vi "CPU_core.vi"(11 "registers":T1 {"P" format="%08b"; "PC" format="%04x"; "SP" format="%02x"; "Y" format="%02x"; "X" format="%02x"; "A" format="%02x"}) -> (1 "clock ticks":u32, 2 "error":bool, 3 "registers":T1 {"P" format="%08b"; "PC" format="%04x"; "SP" format="%02x"; "Y" format="%02x"; "X" format="%02x"; "A" format="%02x"})   [LabVIEW 2018]
uses:
  CPU_registers.ctl
panel:
  # "This 6502 CPU core implements the full set of documented instructions,\ncovering arithmetic (ADC, SBC), logic (AND, ORA, EOR, BIT), shifts and rotates\n(ASL, LSR, ROL, ROR), comparisons (CMP, CPX, CPY), increments/decrements,\nbranches (BPL, BMI, BVC, BVS, BCC, BCS, BNE, BEQ), stack operations (PHA, PLA,\nPHP, PLP, RTS, RTI, BRK, JSR), transfers (TAX, TXA, TAY, TYA, TSX, TXS),\nand memory access (LDA, STA, LDX, STX, LDY, STY) across all addressing modes."
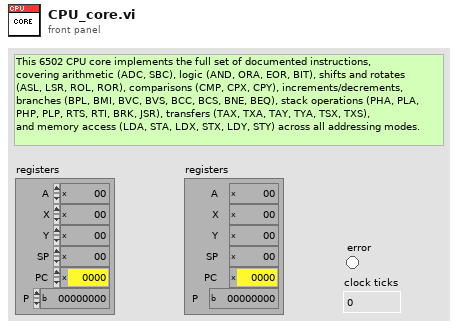
[diagram p1: front panel]
types:
  T1 = typedef "CPU_registers.ctl" = cluster{"A":u8, "X":u8, "Y":u8, "SP":u8, "PC":u16, "P":u8}
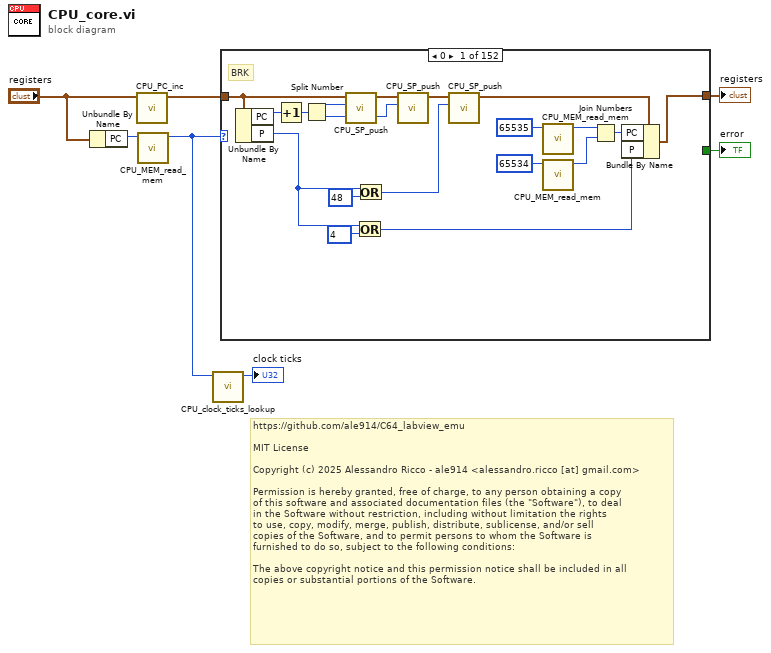
[diagram p0: block diagram]
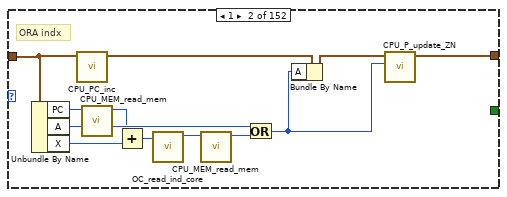
[diagram p2: hidden frame]
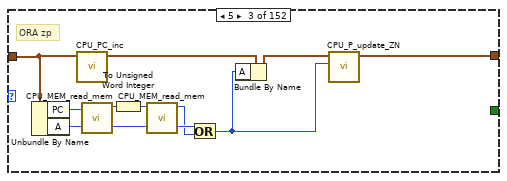
[diagram p3: hidden frame]
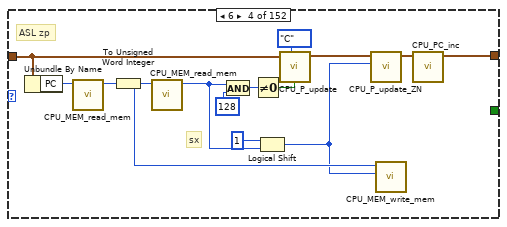
[diagram p4: hidden frame]
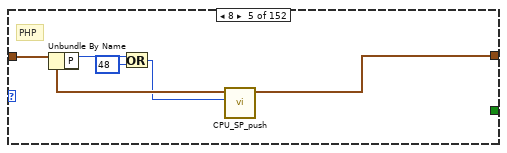
[diagram p5: hidden frame]
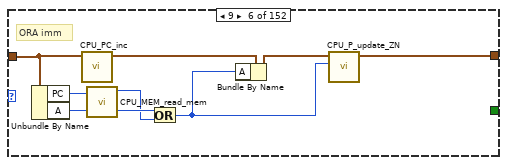
[diagram p6: hidden frame]
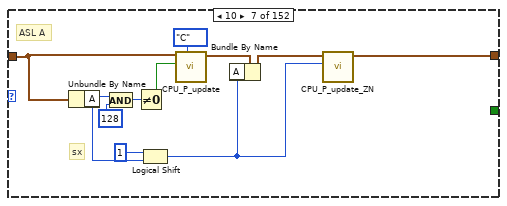
[diagram p7: hidden frame]
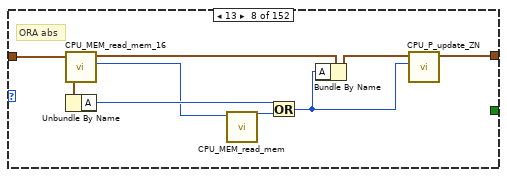
[diagram p8: hidden frame]
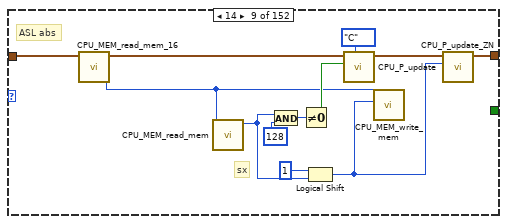
[diagram p9: hidden frame]
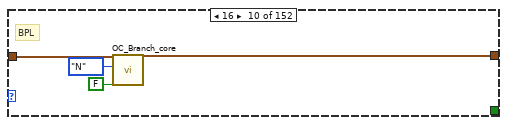
[diagram p10: hidden frame]
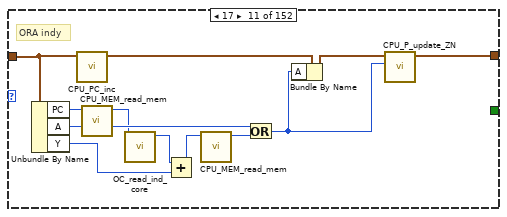
[diagram p11: hidden frame]
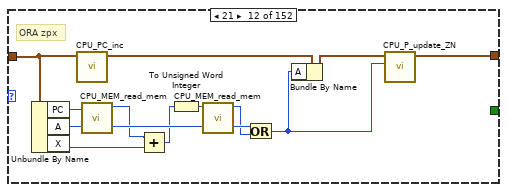
[diagram p12: hidden frame]
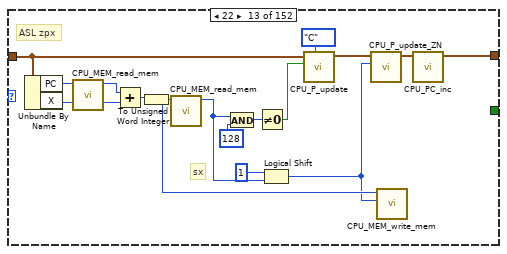
[diagram p13: hidden frame]
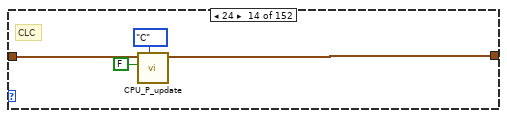
[diagram p14: hidden frame]
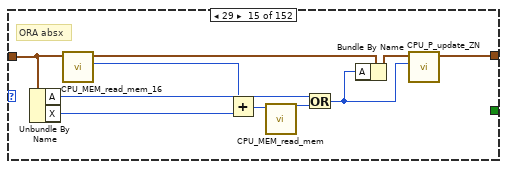
[diagram p15: hidden frame]
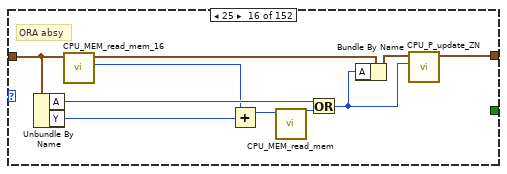
[diagram p16: hidden frame]
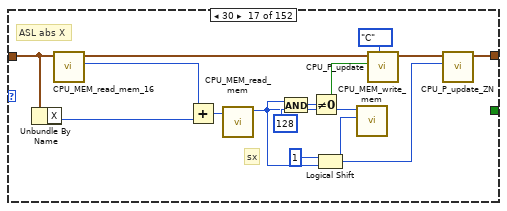
[diagram p17: hidden frame]
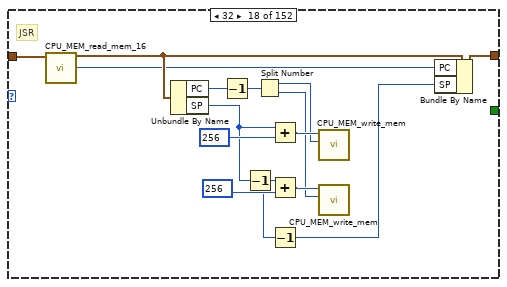
[diagram p18: hidden frame]
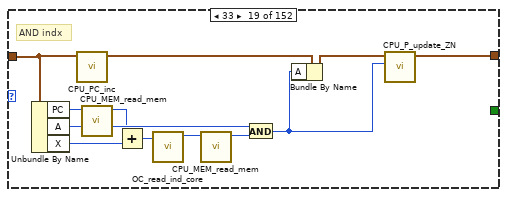
[diagram p19: hidden frame]
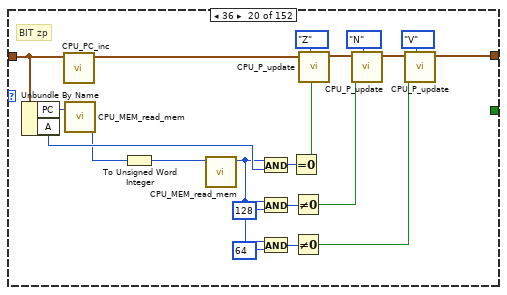
[diagram p20: hidden frame]
diagram:
  # "https://github.com/ale914/C64_labview_emu\n\nMIT License\n\nCopyright (c) 2025 Alessandro Ricco - ale914 <alessandro.ricco [at] gmail.com>\n\nPermission is hereby granted, free of charge, to any person obtaining a copy\nof this software and associated documentation files (the \"Software\"), to deal\nin the Software without restriction, including without limitation the rights\nto use, copy, modify, merge, publish, distribute, sublicense, and/or sell\ncopies of the Software, and to permit persons to whom the Software is\nfurnished to do so, subject to the following conditions:\n\nThe above copyright notice and this permission notice shall be included in all\ncopies or substantial portions of the Software."
  n1 = Unbundle By Name("registers") -> ("PC"=w4:u16)
  n2 = call "CPU_PC_inc.vi"("registers"="registers") -> ("registers"=w7:T1)  [unwired: 10 in]
  n3 = call "CPU_MEM_read_mem.vi"("address"=w4) -> ("value out"=w5:u8)  [unwired: 10 in]
  n4 = call "CPU_clock_ticks_lookup.vi"("opcode"=w5) -> ("clock ticks"=→"clock ticks":u32)  [unwired: 10 in]
  n5 = case shown="0" w5 {
    selector: w5 -> [_ _ _ _ _ _ _ _ _ _ _ _ _ _ _ _ _ _ _ _ _ _ _ _ _ _ _ _ _ _ _ _ _ _ _ _ _ _ _ _ _ _ _ _ _ _ _ _ _ _ _ _ _ _ _ _ _ _ _ _ _ _ _ _ _ _ _ _ _ _ _ _ _ _ _ _ _ _ _ _ _ _ _ _ _ _ _ _ _ _ _ _ _ _ _ _ _ _ _ _ _ _ _ _ _ _ _ _ _ _ _ _ _ _ _ _ _ _ _ _ _ _ _ _ _ _ _ _ _ _ _ _ _ _ _ _ _ _ _ _ _ _ _ _ _ _ _ _ _ _ _ w1390]
    tunnel: w7 -> [w14 w37 w46 w51 w65 w68 w85 w89 w97 w108 w121 w132 w140 w152 w157 w167 w177 w191 w214 w235 w244 w249 w268 w274 w284 w300 w319 w327 w343 w356 w367 w375 w394 w397 w407 w417 w440 w453 w462 w468 w480 w482 w499 w503 w507 w515 w526 w539 w550 w559 w572 w575 w585 w595 w610 w628 w634 w643 w647 w668 w674 w677 w696 w704 w709 w716 w723 w741 w752 w758 w779 w782 w808 w813 w819 w825 w831 w835 w838 w842 w846 w849 w859 w866 w874 w882 w887 w890 w896 w899 w907 w917 w923 w931 w939 w947 w952 w957 w962 w965 w971 w977 w982 w993 w1003 w1013 w1023 w1028 w1031 w1040 w1043 w1051 w1059 w1065 w1087 w1099 w1111 w1115 w1126 w1127 w1141 w1144 w1154 w1164 w1170 w1185 w1199 w1206 w1213 w1220 w1230 w1242 w1249 w1267 w1278 w1285 w1294 w1296 w1309 w1313 w1315 w1318 w1328 w1333 w1340 w1347 w1354 w1363 w1367 w1376 w1381 w1388]
    tunnel: [w23 w34 w43 w62 w64 w71 w78 w92 w101 w107 w118 w129 w150 w151 w162 w172 w183 w203 w211 w231 w241 w265 w273 w277 w282 w313 w322 w328 w342 w353 w364 w390 w391 w402 w412 w420 w441 w450 w459 w478 w479 w485 w493 w504 w510 w519 w525 w536 w547 w568 w569 w580 w590 w601 w609 w621 w632 w641 w665 w669 w672 w680 w699 w706 w713 w720 w727 w740 w749 w775 w776 w788 w803 w811 w817 w823 w827 w832 w837 w841 w845 w848 w854 w864 w872 w880 w884 w889 w894 w898 w904 w915 w920 w929 w937 w945 w949 w954 w959 w967 w973 w979 w981 w991 w1001 w1011 w1021 w1025 w1035 w1037 w1047 w1055 w1063 w1068 w1081 w1093 w1105 w1113 w1122 w1130 w1137 w1147 w1157 w1168 w1169 w1179 w1193 w1204 w1212 w1227 w1235 w1248 w1252 w1260 w1272 w1283 w1292 w1304 w1305 w1311 w1315 w1321 w1330 w1337 w1344 w1349 w1353 w1360 w1374 w1375 w1383 w1388] -> w3
    tunnel: [_ _ _ _ _ _ _ _ _ _ _ _ _ _ _ _ _ _ _ _ _ _ _ _ _ _ _ _ _ _ _ _ _ _ _ _ _ _ _ _ _ _ _ _ _ _ _ _ _ _ _ _ _ _ _ _ _ _ _ _ _ _ _ _ _ _ _ _ _ _ _ _ _ _ _ _ _ _ _ _ _ _ _ _ _ _ _ _ _ _ _ _ _ _ _ _ _ _ _ _ _ _ _ _ _ _ _ _ _ _ _ _ _ _ _ _ _ _ _ _ _ _ _ _ _ _ _ _ _ _ _ _ _ _ _ _ _ _ _ _ _ _ _ _ _ _ _ _ _ _ _ TRUE] -> w2
    frame 0 {
      # "BRK"
      n6 = Unbundle By Name(w14) -> ("PC"=w26:u16, "P"=w16:u8)
      n7 = Increment(x=w26) -> (x+1=w25:u16)
      n8 = Split Number(x=w25) -> (hi(x)=w13:u8, lo(x)=w11:u8)
      n9 = call "CPU_SP_push.vi"("value"=w13, "registers"=w14) -> ("registers"=w12:T1)  [unwired: 9 in]
      n10 = Or(x=w16, y=u8 4) -> (x .or. y?=w15:u8)
      n11 = Or(x=w16, y=u8 48) -> (x .or. y?=w9:u8)
      n12 = call "CPU_SP_push.vi"("value"=w11, "registers"=w12) -> ("registers"=w10:T1)  [unwired: 9 in]
      n13 = call "CPU_SP_push.vi"("value"=w9, "registers"=w10) -> ("registers"=w8:T1)  [unwired: 9 in]
      n14 = call "CPU_MEM_read_mem.vi"("address"=u16 65535) -> ("value out"=w20:u8)  [unwired: 10 in]
      n15 = call "CPU_MEM_read_mem.vi"("address"=u16 65534) -> ("value out"=w19:u8)  [unwired: 10 in]
      n16 = Join Numbers(hi=w20, lo=w19) -> ((hi.lo)=w18:u16)
      n17 = Bundle By Name(cluster=w8, "PC"=w18, "P"=w15) -> (w23:T1)
    }
    frame 1 {
      # "ORA indx"
      n18 = Unbundle By Name(w37) -> ("PC"=w31:u16, "A"=w36:u8, "X"=w32:u8)
      n19 = call "CPU_PC_inc.vi"("registers"=w37) -> ("registers"=w38:T1)  [unwired: 10 in]
      n20 = call "CPU_MEM_read_mem.vi"("address"=w31) -> ("value out"=w30:u8)  [unwired: 10 in]
      n21 = Add(x=w30, y=w32) -> (x+y=w29:u8)
      n22 = call "OC_read_ind_core.vi"("base"=w29) -> ("addr"=w28:u16)  [unwired: 10 in]
      n23 = call "CPU_MEM_read_mem.vi"("address"=w28) -> ("value out"=w27:u8)  [unwired: 10 in]
      n24 = Or(x=w36, y=w27) -> (x .or. y?=w33:u8)
      n25 = Bundle By Name(cluster=w38, "A"=w33) -> (w35:T1)
      n26 = call "CPU_P_update_ZN.vi"("value"=w33, "registers"=w35) -> ("registers"=w34:T1)  [unwired: 9 in]
    }
    frame 5 {
      # "ORA zp"
      n27 = Unbundle By Name(w46) -> ("PC"=w47:u16, "A"=w45:u8)
      n28 = call "CPU_PC_inc.vi"("registers"=w46) -> ("registers"=w48:T1)  [unwired: 10 in]
      n29 = call "CPU_MEM_read_mem.vi"("address"=w47) -> ("value out"=w40:u8)  [unwired: 10 in]
      n30 = To Unsigned Word Integer(number=w40) -> (unsigned 16bit integer=w39:u16)
      n31 = call "CPU_MEM_read_mem.vi"("address"=w39) -> ("value out"=w41:u8)  [unwired: 10 in]
      n32 = Or(x=w45, y=w41) -> (x .or. y?=w42:u8)
      n33 = Bundle By Name(cluster=w48, "A"=w42) -> (w44:T1)
      n34 = call "CPU_P_update_ZN.vi"("value"=w42, "registers"=w44) -> ("registers"=w43:T1)  [unwired: 9 in]
    }
    frame 6 {
      # "sx"
      # "ASL zp"
      n35 = Unbundle By Name(w51) -> ("PC"=w54:u16)
      n36 = call "CPU_MEM_read_mem.vi"("address"=w54) -> ("value out"=w53:u8)  [unwired: 10 in]
      n37 = To Unsigned Word Integer(number=w53) -> (unsigned 16bit integer=w50:u16)
      n38 = call "CPU_MEM_read_mem.vi"("address"=w50) -> ("value out"=w52:u8)  [unwired: 10 in]
      n39 = And(x=w52, y=u8 128 ("base")) -> (x .and. y?=w59:u8)
      n40 = Not Equal To 0?(x=w59) -> (x != 0?=w58:bool)
      n41 = Logical Shift(y=i16 1, x=w52) -> (x << y=w49:u8)
      n42 = call "CPU_P_update.vi"("flag"=enum8{"C", "Z", "I", "D", "B", "V", "N"}."C", "Value"=w58, "registers"=w51) -> ("registers"=w56:T1)  [unwired: 8 in]
      n43 = call "CPU_P_update_ZN.vi"("value"=w49, "registers"=w56) -> ("registers"=w55:T1)  [unwired: 9 in]
      n44 = call "CPU_MEM_write_mem.vi"("value"=w49, "address"=w50) -> ()  [unwired: 10 in]
      n45 = call "CPU_PC_inc.vi"("registers"=w55) -> ("registers"=w62:T1)  [unwired: 10 in]
    }
    frame 8 {
      # "PHP"
      n46 = Unbundle By Name(w65) -> ("P"=w66:u8)
      n47 = Or(x=w66, y=u8 48) -> (x .or. y?=w63:u8)
      n48 = call "CPU_SP_push.vi"("value"=w63, "registers"=w65) -> ("registers"=w64:T1)  [unwired: 9 in]
    }
    frame 9 {
      # "ORA imm"
      n49 = Unbundle By Name(w68) -> ("PC"=w75:u16, "A"=w74:u8)
      n50 = call "CPU_PC_inc.vi"("registers"=w68) -> ("registers"=w69:T1)  [unwired: 10 in]
      n51 = call "CPU_MEM_read_mem.vi"("address"=w75) -> ("value out"=w73:u8)  [unwired: 10 in]
      n52 = Or(x=w74, y=w73) -> (x .or. y?=w70:u8)
      n53 = Bundle By Name(cluster=w69, "A"=w70) -> (w72:T1)
      n54 = call "CPU_P_update_ZN.vi"("value"=w70, "registers"=w72) -> ("registers"=w71:T1)  [unwired: 9 in]
    }
    frame 10 {
      # "sx"
      # "ASL A"
      n55 = Unbundle By Name(w85) -> ("A"=w81:u8)
      n56 = And(x=w81, y=u8 128 ("base")) -> (x .and. y?=w83:u8)
      n57 = Not Equal To 0?(x=w83) -> (x != 0?=w82:bool)
      n58 = Logical Shift(y=i16 1, x=w81) -> (x << y=w76:u8)
      n59 = call "CPU_P_update.vi"("flag"=enum8{"C", "Z", "I", "D", "B", "V", "N"}."C", "Value"=w82, "registers"=w85) -> ("registers"=w79:T1)  [unwired: 8 in]
      n60 = Bundle By Name(cluster=w79, "A"=w76) -> (w77:T1)
      n61 = call "CPU_P_update_ZN.vi"("value"=w76, "registers"=w77) -> ("registers"=w78:T1)  [unwired: 9 in]
    }
    frame 13 {
      # "ORA abs"
      n62 = call "CPU_MEM_read_mem_16.vi"("registers"=w89) -> ("value"=w87:u16, "registers"=w88:T1)  [unwired: 9 in]
      n63 = Unbundle By Name(w89) -> ("A"=w94:u8)
      n64 = call "CPU_MEM_read_mem.vi"("address"=w87) -> ("value out"=w90:u8)  [unwired: 10 in]
      n65 = Or(x=w94, y=w90) -> (x .or. y?=w91:u8)
      n66 = Bundle By Name(cluster=w88, "A"=w91) -> (w93:T1)
      n67 = call "CPU_P_update_ZN.vi"("value"=w91, "registers"=w93) -> ("registers"=w92:T1)  [unwired: 9 in]
    }
    frame 14 {
      # "sx"
      # "ASL abs"
      n68 = call "CPU_MEM_read_mem_16.vi"("registers"=w97) -> ("value"=w95:u16, "registers"=w96:T1)  [unwired: 9 in]
      n69 = call "CPU_MEM_read_mem.vi"("address"=w95) -> ("value out"=w100:u8)  [unwired: 10 in]
      n70 = And(x=w100, y=u8 128 ("base")) -> (x .and. y?=w104:u8)
      n71 = Not Equal To 0?(x=w104) -> (x != 0?=w103:bool)
      n72 = Logical Shift(y=i16 1, x=w100) -> (x << y=w98:u8)
      n73 = call "CPU_P_update.vi"("flag"=enum8{"C", "Z", "I", "D", "B", "V", "N"}."C", "Value"=w103, "registers"=w96) -> ("registers"=w99:T1)  [unwired: 8 in]
      n74 = call "CPU_MEM_write_mem.vi"("value"=w98, "address"=w95) -> ()  [unwired: 10 in]
      n75 = call "CPU_P_update_ZN.vi"("value"=w98, "registers"=w99) -> ("registers"=w101:T1)  [unwired: 9 in]
    }
    frame 16 {
      # "BPL"
      n76 = call "OC_Branch_core.vi"("if set/clear"=FALSE, "flag"=enum8{"C", "Z", "I", "D", "B", "V", "N"}."N", "registers"=w108) -> ("registers"=w107:T1)  [unwired: 8 in]
    }
    frame 17 {
      # "ORA indy"
      n77 = Unbundle By Name(w121) -> ("PC"=w116:u16, "A"=w120:u8, "Y"=w112:u8)
      n78 = call "CPU_PC_inc.vi"("registers"=w121) -> ("registers"=w122:T1)  [unwired: 10 in]
      n79 = call "CPU_MEM_read_mem.vi"("address"=w116) -> ("value out"=w114:u8)  [unwired: 10 in]
      n80 = call "OC_read_ind_core.vi"("base"=w114) -> ("addr"=w113:u16)  [unwired: 10 in]
      n81 = Add(x=w113, y=w112) -> (x+y=w111:u16)
      n82 = call "CPU_MEM_read_mem.vi"("address"=w111) -> ("value out"=w115:u8)  [unwired: 10 in]
      n83 = Or(x=w120, y=w115) -> (x .or. y?=w117:u8)
      n84 = Bundle By Name(cluster=w122, "A"=w117) -> (w119:T1)
      n85 = call "CPU_P_update_ZN.vi"("value"=w117, "registers"=w119) -> ("registers"=w118:T1)  [unwired: 9 in]
    }
    frame 21 {
      # "ORA zpx"
      n86 = Unbundle By Name(w132) -> ("PC"=w133:u16, "A"=w131:u8, "X"=w126:u8)
      n87 = call "CPU_PC_inc.vi"("registers"=w132) -> ("registers"=w134:T1)  [unwired: 10 in]
      n88 = call "CPU_MEM_read_mem.vi"("address"=w133) -> ("value out"=w124:u8)  [unwired: 10 in]
      n89 = Add(x=w124, y=w126) -> (x+y=w125:u8)
      n90 = To Unsigned Word Integer(number=w125) -> (unsigned 16bit integer=w123:u16)
      n91 = call "CPU_MEM_read_mem.vi"("address"=w123) -> ("value out"=w127:u8)  [unwired: 10 in]
      n92 = Or(x=w131, y=w127) -> (x .or. y?=w128:u8)
      n93 = Bundle By Name(cluster=w134, "A"=w128) -> (w130:T1)
      n94 = call "CPU_P_update_ZN.vi"("value"=w128, "registers"=w130) -> ("registers"=w129:T1)  [unwired: 9 in]
    }
    frame 22 {
      # "sx"
      # "ASL zpx"
      n95 = Unbundle By Name(w140) -> ("PC"=w142:u16, "X"=w137:u8)
      n96 = call "CPU_MEM_read_mem.vi"("address"=w142) -> ("value out"=w136:u8)  [unwired: 10 in]
      n97 = Add(x=w136, y=w137) -> (x+y=w135:u8)
      n98 = To Unsigned Word Integer(number=w135) -> (unsigned 16bit integer=w139:u16)
      n99 = call "CPU_MEM_read_mem.vi"("address"=w139) -> ("value out"=w141:u8)  [unwired: 10 in]
      n100 = And(x=w141, y=u8 128 ("base")) -> (x .and. y?=w147:u8)
      n101 = Not Equal To 0?(x=w147) -> (x != 0?=w146:bool)
      n102 = Logical Shift(y=i16 1, x=w141) -> (x << y=w138:u8)
      n103 = call "CPU_P_update.vi"("flag"=enum8{"C", "Z", "I", "D", "B", "V", "N"}."C", "Value"=w146, "registers"=w140) -> ("registers"=w144:T1)  [unwired: 8 in]
      n104 = call "CPU_P_update_ZN.vi"("value"=w138, "registers"=w144) -> ("registers"=w143:T1)  [unwired: 9 in]
      n105 = call "CPU_MEM_write_mem.vi"("value"=w138, "address"=w139) -> ()  [unwired: 10 in]
      n106 = call "CPU_PC_inc.vi"("registers"=w143) -> ("registers"=w150:T1)  [unwired: 10 in]
    }
    frame 24 {
      # "CLC"
      n107 = call "CPU_P_update.vi"("flag"=enum8{"C", "Z", "I", "D", "B", "V", "N"}."C", "Value"=FALSE, "registers"=w152) -> ("registers"=w151:T1)  [unwired: 8 in]
    }
    frame 29 {
      # "ORA absx"
      n108 = Unbundle By Name(w157) -> ("A"=w164:u8, "X"=w158:u8)
      n109 = call "CPU_MEM_read_mem_16.vi"("registers"=w157) -> ("value"=w155:u16, "registers"=w156:T1)  [unwired: 9 in]
      n110 = Add(x=w155, y=w158) -> (x+y=w159:u16)
      n111 = call "CPU_MEM_read_mem.vi"("address"=w159) -> ("value out"=w160:u8)  [unwired: 10 in]
      n112 = Or(x=w164, y=w160) -> (x .or. y?=w161:u8)
      n113 = Bundle By Name(cluster=w156, "A"=w161) -> (w163:T1)
      n114 = call "CPU_P_update_ZN.vi"("value"=w161, "registers"=w163) -> ("registers"=w162:T1)  [unwired: 9 in]
    }
    frame 25 {
      # "ORA absy"
      n115 = Unbundle By Name(w167) -> ("A"=w174:u8, "Y"=w168:u8)
      n116 = call "CPU_MEM_read_mem_16.vi"("registers"=w167) -> ("value"=w165:u16, "registers"=w166:T1)  [unwired: 9 in]
      n117 = Add(x=w165, y=w168) -> (x+y=w169:u16)
      n118 = call "CPU_MEM_read_mem.vi"("address"=w169) -> ("value out"=w170:u8)  [unwired: 10 in]
      n119 = Or(x=w174, y=w170) -> (x .or. y?=w171:u8)
      n120 = Bundle By Name(cluster=w166, "A"=w171) -> (w173:T1)
      n121 = call "CPU_P_update_ZN.vi"("value"=w171, "registers"=w173) -> ("registers"=w172:T1)  [unwired: 9 in]
    }
    frame 30 {
      # "sx"
      # "ASL abs X"
      n122 = Unbundle By Name(w177) -> ("X"=w178:u8)
      n123 = call "CPU_MEM_read_mem_16.vi"("registers"=w177) -> ("value"=w175:u16, "registers"=w176:T1)  [unwired: 9 in]
      n124 = Add(x=w175, y=w178) -> (x+y=w179:u16)
      n125 = call "CPU_MEM_read_mem.vi"("address"=w179) -> ("value out"=w182:u8)  [unwired: 10 in]
      n126 = And(x=w182, y=u8 128 ("base")) -> (x .and. y?=w186:u8)
      n127 = Not Equal To 0?(x=w186) -> (x != 0?=w185:bool)
      n128 = Logical Shift(y=i16 1, x=w182) -> (x << y=w180:u8)
      n129 = call "CPU_MEM_write_mem.vi"("value"=w180, "address"=w179) -> ()  [unwired: 10 in]
      n130 = call "CPU_P_update.vi"("flag"=enum8{"C", "Z", "I", "D", "B", "V", "N"}."C", "Value"=w185, "registers"=w176) -> ("registers"=w181:T1)  [unwired: 8 in]
      n131 = call "CPU_P_update_ZN.vi"("value"=w180, "registers"=w181) -> ("registers"=w183:T1)  [unwired: 9 in]
    }
    frame 32 {
      # "JSR"
      n132 = call "CPU_MEM_read_mem_16.vi"("registers"=w191) -> ("value"=w189:u16, "registers"=w190:T1)  [unwired: 9 in]
      n133 = Unbundle By Name(w190) -> ("PC"=w193:u16, "SP"=w196:u8)
      n134 = Decrement(x=w193) -> (x-1=w192:u16)
      n135 = Decrement(x=w196) -> (x-1=w195:u8)
      n136 = Split Number(x=w192) -> (hi(x)=w200:u8, lo(x)=w197:u8)
      n137 = Add(x=w196, y=u16 256) -> (x+y=w201:u16)
      n138 = Add(x=w195, y=u16 256) -> (x+y=w199:u16)
      n139 = Decrement(x=w195) -> (x-1=w194:u8)
      n140 = call "CPU_MEM_write_mem.vi"("value"=w200, "address"=w201) -> ()  [unwired: 10 in]
      n141 = call "CPU_MEM_write_mem.vi"("value"=w197, "address"=w199) -> ()  [unwired: 10 in]
      n142 = Bundle By Name(cluster=w190, "PC"=w189, "SP"=w194) -> (w203:T1)
    }
    frame 33 {
      # "AND indx"
      n143 = Unbundle By Name(w214) -> ("PC"=w208:u16, "A"=w213:u8, "X"=w209:u8)
      n144 = call "CPU_PC_inc.vi"("registers"=w214) -> ("registers"=w215:T1)  [unwired: 10 in]
      n145 = call "CPU_MEM_read_mem.vi"("address"=w208) -> ("value out"=w207:u8)  [unwired: 10 in]
      n146 = Add(x=w207, y=w209) -> (x+y=w206:u8)
      n147 = call "OC_read_ind_core.vi"("base"=w206) -> ("addr"=w205:u16)  [unwired: 10 in]
      n148 = call "CPU_MEM_read_mem.vi"("address"=w205) -> ("value out"=w204:u8)  [unwired: 10 in]
      n149 = And(x=w213, y=w204) -> (x .and. y?=w210:u8)
      n150 = Bundle By Name(cluster=w215, "A"=w210) -> (w212:T1)
      n151 = call "CPU_P_update_ZN.vi"("value"=w210, "registers"=w212) -> ("registers"=w211:T1)  [unwired: 9 in]
    }
    frame 36 {
      # "BIT zp"
      n152 = Unbundle By Name(w235) -> ("PC"=w236:u16, "A"=w228:u8)
      n153 = call "CPU_PC_inc.vi"("registers"=w235) -> ("registers"=w218:T1)  [unwired: 10 in]
      n154 = call "CPU_MEM_read_mem.vi"("address"=w236) -> ("value out"=w217:u8)  [unwired: 10 in]
      n155 = To Unsigned Word Integer(number=w217) -> (unsigned 16bit integer=w216:u16)
      n156 = call "CPU_MEM_read_mem.vi"("address"=w216) -> ("value out"=w220:u8)  [unwired: 10 in]
      n157 = And(x=w220, y=w228) -> (x .and. y?=w227:u8)
      n158 = And(x=w220, y=u8 128 ("base")) -> (x .and. y?=w224:u8)
      n159 = And(x=w220, y=u8 64 ("base")) -> (x .and. y?=w222:u8)
      n160 = Equal To 0?(x=w227) -> (x = 0?=w226:bool)
      n161 = Not Equal To 0?(x=w224) -> (x != 0?=w223:bool)
      n162 = Not Equal To 0?(x=w222) -> (x != 0?=w219:bool)
      n163 = call "CPU_P_update.vi"("flag"=enum8{"C", "Z", "I", "D", "B", "V", "N"}."Z", "Value"=w226, "registers"=w218) -> ("registers"=w229:T1)  [unwired: 8 in]
      n164 = call "CPU_P_update.vi"("flag"=enum8{"C", "Z", "I", "D", "B", "V", "N"}."N", "Value"=w223, "registers"=w229) -> ("registers"=w230:T1)  [unwired: 8 in]
      n165 = call "CPU_P_update.vi"("flag"=enum8{"C", "Z", "I", "D", "B", "V", "N"}."V", "Value"=w219, "registers"=w230) -> ("registers"=w231:T1)  [unwired: 8 in]
    }
    frame 37 {
      # "AND zp"
      n166 = Unbundle By Name(w244) -> ("PC"=w245:u16, "A"=w243:u8)
      n167 = call "CPU_PC_inc.vi"("registers"=w244) -> ("registers"=w246:T1)  [unwired: 10 in]
      n168 = call "CPU_MEM_read_mem.vi"("address"=w245) -> ("value out"=w238:u8)  [unwired: 10 in]
      n169 = To Unsigned Word Integer(number=w238) -> (unsigned 16bit integer=w237:u16)
      n170 = call "CPU_MEM_read_mem.vi"("address"=w237) -> ("value out"=w239:u8)  [unwired: 10 in]
      n171 = And(x=w243, y=w239) -> (x .and. y?=w240:u8)
      n172 = Bundle By Name(cluster=w246, "A"=w240) -> (w242:T1)
      n173 = call "CPU_P_update_ZN.vi"("value"=w240, "registers"=w242) -> ("registers"=w241:T1)  [unwired: 9 in]
    }
    frame 38 {
      # "sx"
      # "ROL zp"
      n174 = Unbundle By Name(w249) -> ("PC"=w259:u16)
      n175 = call "CPU_MEM_read_mem.vi"("address"=w259) -> ("value out"=w258:u8)  [unwired: 10 in]
      n176 = To Unsigned Word Integer(number=w258) -> (unsigned 16bit integer=w251:u16)
      n177 = call "CPU_MEM_read_mem.vi"("address"=w251) -> ("value out"=w257:u8)  [unwired: 10 in]
      n178 = call "CPU_P_get_flag.vi"("flag"=enum8{"C", "Z", "I", "D", "B", "V", "N"}."C", "registers"=w249) -> ("Value"=w255:bool)  [unwired: 8 in, 1 out]
      n179 = And(x=w257, y=u8 128 ("base")) -> (x .and. y?=w262:u8)
      n180 = Boolean To (0,1)(Boolean=w255) -> (0, 1=w254:i16)
      n181 = Not Equal To 0?(x=w262) -> (x != 0?=w261:bool)
      n182 = Logical Shift(y=i16 1, x=w257) -> (x << y=w252:u8)
      n183 = To Unsigned Byte Integer(number=w254) -> (unsigned 8bit integer=w253:u8)
      n184 = Or(x=w252, y=w253) -> (x .or. y?=w250:u8)
      n185 = call "CPU_P_update_ZN.vi"("value"=w250, "registers"=w249) -> ("registers"=w248:T1)  [unwired: 9 in]
      n186 = call "CPU_MEM_write_mem.vi"("value"=w250, "address"=w251) -> ()  [unwired: 10 in]
      n187 = call "CPU_P_update.vi"("flag"=enum8{"C", "Z", "I", "D", "B", "V", "N"}."C", "Value"=w261, "registers"=w248) -> ("registers"=w247:T1)  [unwired: 8 in]
      n188 = call "CPU_PC_inc.vi"("registers"=w247) -> ("registers"=w265:T1)  [unwired: 10 in]
    }
    frame 40 {
      # "PLP"
      n189 = call "CPU_SP_pop.vi"("registers"=w268) -> ("value"=w266:u8, "registers"=w267:T1)  [unwired: 9 in]
      n190 = And(x=w266, y=u8 239) -> (x .and. y?=w271:u8)
      n191 = Or(x=w271, y=u8 32) -> (x .or. y?=w270:u8)
      n192 = Bundle By Name(cluster=w267, "P"=w270) -> (w273:T1)
    }
    frame 41 {
      # "AND imm"
      n193 = Unbundle By Name(w274) -> ("PC"=w281:u16, "A"=w280:u8)
      n194 = call "CPU_MEM_read_mem.vi"("address"=w281) -> ("value out"=w279:u8)  [unwired: 10 in]
      n195 = call "CPU_PC_inc.vi"("registers"=w274) -> ("registers"=w275:T1)  [unwired: 10 in]
      n196 = And(x=w280, y=w279) -> (x .and. y?=w276:u8)
      n197 = Bundle By Name(cluster=w275, "A"=w276) -> (w278:T1)
      n198 = call "CPU_P_update_ZN.vi"("value"=w276, "registers"=w278) -> ("registers"=w277:T1)  [unwired: 9 in]
    }
    frame 42 {
      # "sx"
      # "ROL A"
      n199 = Unbundle By Name(w284) -> ("A"=w293:u8)
      n200 = call "CPU_P_get_flag.vi"("flag"=enum8{"C", "Z", "I", "D", "B", "V", "N"}."C", "registers"=w284) -> ("Value"=w289:bool)  [unwired: 8 in, 1 out]
      n201 = And(x=w293, y=u8 128 ("base")) -> (x .and. y?=w295:u8)
      n202 = Boolean To (0,1)(Boolean=w289) -> (0, 1=w288:i16)
      n203 = Not Equal To 0?(x=w295) -> (x != 0?=w294:bool)
      n204 = Logical Shift(y=i16 1, x=w293) -> (x << y=w291:u8)
      n205 = To Unsigned Byte Integer(number=w288) -> (unsigned 8bit integer=w287:u8)
      n206 = Or(x=w291, y=w287) -> (x .or. y?=w285:u8)
      n207 = Bundle By Name(cluster=w284, "A"=w285) -> (w286:T1)
      n208 = call "CPU_P_update_ZN.vi"("value"=w285, "registers"=w286) -> ("registers"=w283:T1)  [unwired: 9 in]
      n209 = call "CPU_P_update.vi"("flag"=enum8{"C", "Z", "I", "D", "B", "V", "N"}."C", "Value"=w294, "registers"=w283) -> ("registers"=w282:T1)  [unwired: 8 in]
    }
    frame 44 {
      # "BIT abs"
      n210 = Unbundle By Name(w300) -> ("A"=w310:u8)
      n211 = call "CPU_MEM_read_mem_16.vi"("registers"=w300) -> ("value"=w298:u16, "registers"=w299:T1)  [unwired: 9 in]
      n212 = call "CPU_MEM_read_mem.vi"("address"=w298) -> ("value out"=w302:u8)  [unwired: 10 in]
      n213 = And(x=w310, y=w302) -> (x .and. y?=w309:u8)
      n214 = And(x=w302, y=u8 128 ("base")) -> (x .and. y?=w306:u8)
      n215 = And(x=w302, y=u8 64 ("base")) -> (x .and. y?=w304:u8)
      n216 = Equal To 0?(x=w309) -> (x = 0?=w308:bool)
      n217 = Not Equal To 0?(x=w306) -> (x != 0?=w305:bool)
      n218 = Not Equal To 0?(x=w304) -> (x != 0?=w301:bool)
      n219 = call "CPU_P_update.vi"("flag"=enum8{"C", "Z", "I", "D", "B", "V", "N"}."Z", "Value"=w308, "registers"=w299) -> ("registers"=w311:T1)  [unwired: 8 in]
      n220 = call "CPU_P_update.vi"("flag"=enum8{"C", "Z", "I", "D", "B", "V", "N"}."N", "Value"=w305, "registers"=w311) -> ("registers"=w312:T1)  [unwired: 8 in]
      n221 = call "CPU_P_update.vi"("flag"=enum8{"C", "Z", "I", "D", "B", "V", "N"}."V", "Value"=w301, "registers"=w312) -> ("registers"=w313:T1)  [unwired: 8 in]
    }
    frame 45 {
      # "AND abs"
      n222 = Unbundle By Name(w319) -> ("A"=w324:u8)
      n223 = call "CPU_MEM_read_mem_16.vi"("registers"=w319) -> ("value"=w317:u16, "registers"=w318:T1)  [unwired: 9 in]
      n224 = call "CPU_MEM_read_mem.vi"("address"=w317) -> ("value out"=w320:u8)  [unwired: 10 in]
      n225 = And(x=w324, y=w320) -> (x .and. y?=w321:u8)
      n226 = Bundle By Name(cluster=w318, "A"=w321) -> (w323:T1)
      n227 = call "CPU_P_update_ZN.vi"("value"=w321, "registers"=w323) -> ("registers"=w322:T1)  [unwired: 9 in]
    }
    frame 46 {
      # "sx"
      # "ROL abs"
      n228 = call "CPU_MEM_read_mem_16.vi"("registers"=w327) -> ("value"=w325:u16, "registers"=w326:T1)  [unwired: 9 in]
      n229 = call "CPU_MEM_read_mem.vi"("address"=w325) -> ("value out"=w329:u8)  [unwired: 10 in]
      n230 = call "CPU_P_get_flag.vi"("flag"=enum8{"C", "Z", "I", "D", "B", "V", "N"}."C", "registers"=w327) -> ("Value"=w335:bool)  [unwired: 8 in, 1 out]
      n231 = Boolean To (0,1)(Boolean=w335) -> (0, 1=w334:i16)
      n232 = And(x=w329, y=u8 128 ("base")) -> (x .and. y?=w339:u8)
      n233 = Logical Shift(y=i16 1, x=w329) -> (x << y=w332:u8)
      n234 = To Unsigned Byte Integer(number=w334) -> (unsigned 8bit integer=w333:u8)
      n235 = Not Equal To 0?(x=w339) -> (x != 0?=w338:bool)
      n236 = Or(x=w332, y=w333) -> (x .or. y?=w331:u8)
      n237 = call "CPU_P_update_ZN.vi"("value"=w331, "registers"=w326) -> ("registers"=w330:T1)  [unwired: 9 in]
      n238 = call "CPU_MEM_write_mem.vi"("value"=w331, "address"=w325) -> ()  [unwired: 10 in]
      n239 = call "CPU_P_update.vi"("flag"=enum8{"C", "Z", "I", "D", "B", "V", "N"}."C", "Value"=w338, "registers"=w330) -> ("registers"=w328:T1)  [unwired: 8 in]
    }
    frame 48 {
      # "BMI"
      n240 = call "OC_Branch_core.vi"("if set/clear"=TRUE, "flag"=enum8{"C", "Z", "I", "D", "B", "V", "N"}."N", "registers"=w343) -> ("registers"=w342:T1)  [unwired: 8 in]
    }
    frame 49 {
      # "AND indy"
      n241 = Unbundle By Name(w356) -> ("PC"=w351:u16, "A"=w355:u8, "Y"=w347:u8)
      n242 = call "CPU_PC_inc.vi"("registers"=w356) -> ("registers"=w357:T1)  [unwired: 10 in]
      n243 = call "CPU_MEM_read_mem.vi"("address"=w351) -> ("value out"=w349:u8)  [unwired: 10 in]
      n244 = call "OC_read_ind_core.vi"("base"=w349) -> ("addr"=w348:u16)  [unwired: 10 in]
      n245 = Add(x=w348, y=w347) -> (x+y=w346:u16)
      n246 = call "CPU_MEM_read_mem.vi"("address"=w346) -> ("value out"=w350:u8)  [unwired: 10 in]
      n247 = And(x=w355, y=w350) -> (x .and. y?=w352:u8)
      n248 = Bundle By Name(cluster=w357, "A"=w352) -> (w354:T1)
      n249 = call "CPU_P_update_ZN.vi"("value"=w352, "registers"=w354) -> ("registers"=w353:T1)  [unwired: 9 in]
    }
    frame 53 {
      # "AND zpx"
      n250 = Unbundle By Name(w367) -> ("PC"=w368:u16, "A"=w366:u8, "X"=w361:u8)
      n251 = call "CPU_PC_inc.vi"("registers"=w367) -> ("registers"=w369:T1)  [unwired: 10 in]
      n252 = call "CPU_MEM_read_mem.vi"("address"=w368) -> ("value out"=w359:u8)  [unwired: 10 in]
      n253 = Add(x=w359, y=w361) -> (x+y=w360:u8)
      n254 = To Unsigned Word Integer(number=w360) -> (unsigned 16bit integer=w358:u16)
      n255 = call "CPU_MEM_read_mem.vi"("address"=w358) -> ("value out"=w362:u8)  [unwired: 10 in]
      n256 = And(x=w366, y=w362) -> (x .and. y?=w363:u8)
      n257 = Bundle By Name(cluster=w369, "A"=w363) -> (w365:T1)
      n258 = call "CPU_P_update_ZN.vi"("value"=w363, "registers"=w365) -> ("registers"=w364:T1)  [unwired: 9 in]
    }
    frame 54 {
      # "sx"
      # "ROL zp X"
      n259 = Unbundle By Name(w375) -> ("PC"=w384:u16, "X"=w372:u8)
      n260 = call "CPU_MEM_read_mem.vi"("address"=w384) -> ("value out"=w371:u8)  [unwired: 10 in]
      n261 = Add(x=w371, y=w372) -> (x+y=w370:u8)
      n262 = To Unsigned Word Integer(number=w370) -> (unsigned 16bit integer=w377:u16)
      n263 = call "CPU_MEM_read_mem.vi"("address"=w377) -> ("value out"=w383:u8)  [unwired: 10 in]
      n264 = call "CPU_P_get_flag.vi"("flag"=enum8{"C", "Z", "I", "D", "B", "V", "N"}."C", "registers"=w375) -> ("Value"=w381:bool)  [unwired: 8 in, 1 out]
      n265 = And(x=w383, y=u8 128 ("base")) -> (x .and. y?=w387:u8)
      n266 = Boolean To (0,1)(Boolean=w381) -> (0, 1=w380:i16)
      n267 = Not Equal To 0?(x=w387) -> (x != 0?=w386:bool)
      n268 = Logical Shift(y=i16 1, x=w383) -> (x << y=w378:u8)
      n269 = To Unsigned Byte Integer(number=w380) -> (unsigned 8bit integer=w379:u8)
      n270 = Or(x=w378, y=w379) -> (x .or. y?=w376:u8)
      n271 = call "CPU_P_update_ZN.vi"("value"=w376, "registers"=w375) -> ("registers"=w374:T1)  [unwired: 9 in]
      n272 = call "CPU_P_update.vi"("flag"=enum8{"C", "Z", "I", "D", "B", "V", "N"}."C", "Value"=w386, "registers"=w374) -> ("registers"=w373:T1)  [unwired: 8 in]
      n273 = call "CPU_MEM_write_mem.vi"("value"=w376, "address"=w377) -> ()  [unwired: 10 in]
      n274 = call "CPU_PC_inc.vi"("registers"=w373) -> ("registers"=w390:T1)  [unwired: 10 in]
    }
    frame 56 {
      # "SEC"
      n275 = call "CPU_P_update.vi"("flag"=enum8{"C", "Z", "I", "D", "B", "V", "N"}."C", "Value"=TRUE, "registers"=w394) -> ("registers"=w391:T1)  [unwired: 8 in]
    }
    frame 57 {
      # "AND absy"
      n276 = Unbundle By Name(w397) -> ("A"=w404:u8, "Y"=w398:u8)
      n277 = call "CPU_MEM_read_mem_16.vi"("registers"=w397) -> ("value"=w395:u16, "registers"=w396:T1)  [unwired: 9 in]
      n278 = Add(x=w395, y=w398) -> (x+y=w399:u16)
      n279 = call "CPU_MEM_read_mem.vi"("address"=w399) -> ("value out"=w400:u8)  [unwired: 10 in]
      n280 = And(x=w404, y=w400) -> (x .and. y?=w401:u8)
      n281 = Bundle By Name(cluster=w396, "A"=w401) -> (w403:T1)
      n282 = call "CPU_P_update_ZN.vi"("value"=w401, "registers"=w403) -> ("registers"=w402:T1)  [unwired: 9 in]
    }
    frame 61 {
      # "AND absx"
      n283 = Unbundle By Name(w407) -> ("A"=w414:u8, "X"=w408:u8)
      n284 = call "CPU_MEM_read_mem_16.vi"("registers"=w407) -> ("value"=w405:u16, "registers"=w406:T1)  [unwired: 9 in]
      n285 = Add(x=w405, y=w408) -> (x+y=w409:u16)
      n286 = call "CPU_MEM_read_mem.vi"("address"=w409) -> ("value out"=w410:u8)  [unwired: 10 in]
      n287 = And(x=w414, y=w410) -> (x .and. y?=w411:u8)
      n288 = Bundle By Name(cluster=w406, "A"=w411) -> (w413:T1)
      n289 = call "CPU_P_update_ZN.vi"("value"=w411, "registers"=w413) -> ("registers"=w412:T1)  [unwired: 9 in]
    }
    frame 62 {
      # "sx"
      # "ROL abs X"
      n290 = Unbundle By Name(w417) -> ("X"=w418:u8)
      n291 = call "CPU_MEM_read_mem_16.vi"("registers"=w417) -> ("value"=w415:u16, "registers"=w416:T1)  [unwired: 9 in]
      n292 = Add(x=w415, y=w418) -> (x+y=w419:u16)
      n293 = call "CPU_MEM_read_mem.vi"("address"=w419) -> ("value out"=w421:u8)  [unwired: 10 in]
      n294 = call "CPU_P_get_flag.vi"("flag"=enum8{"C", "Z", "I", "D", "B", "V", "N"}."C", "registers"=w417) -> ("Value"=w427:bool)  [unwired: 8 in, 1 out]
      n295 = Boolean To (0,1)(Boolean=w427) -> (0, 1=w426:i16)
      n296 = And(x=w421, y=u8 128 ("base")) -> (x .and. y?=w431:u8)
      n297 = To Unsigned Byte Integer(number=w426) -> (unsigned 8bit integer=w425:u8)
      n298 = Logical Shift(y=i16 1, x=w421) -> (x << y=w424:u8)
      n299 = Not Equal To 0?(x=w431) -> (x != 0?=w430:bool)
      n300 = Or(x=w424, y=w425) -> (x .or. y?=w423:u8)
      n301 = call "CPU_P_update_ZN.vi"("value"=w423, "registers"=w416) -> ("registers"=w422:T1)  [unwired: 9 in]
      n302 = call "CPU_MEM_write_mem.vi"("value"=w423, "address"=w419) -> ()  [unwired: 10 in]
      n303 = call "CPU_P_update.vi"("flag"=enum8{"C", "Z", "I", "D", "B", "V", "N"}."C", "Value"=w430, "registers"=w422) -> ("registers"=w420:T1)  [unwired: 8 in]
    }
    frame 64 {
      # "RTI"
      n304 = call "CPU_SP_pop.vi"("registers"=w440) -> ("value"=w439:u8, "registers"=w438:T1)  [unwired: 9 in]
      n305 = call "CPU_SP_pop.vi"("registers"=w438) -> ("value"=w436:u8, "registers"=w437:T1)  [unwired: 9 in]
      n306 = call "CPU_SP_pop.vi"("registers"=w437) -> ("value"=w435:u8, "registers"=w434:T1)  [unwired: 9 in]
      n307 = Join Numbers(hi=w435, lo=w436) -> ((hi.lo)=w442:u16)
      n308 = Bundle By Name(cluster=w434, "P"=w439, "PC"=w442) -> (w441:T1)
    }
    frame 65 {
      # "EOR indx"
      n309 = Unbundle By Name(w453) -> ("PC"=w447:u16, "A"=w452:u8, "X"=w448:u8)
      n310 = call "CPU_PC_inc.vi"("registers"=w453) -> ("registers"=w454:T1)  [unwired: 10 in]
      n311 = call "CPU_MEM_read_mem.vi"("address"=w447) -> ("value out"=w446:u8)  [unwired: 10 in]
      n312 = Add(x=w446, y=w448) -> (x+y=w445:u8)
      n313 = call "OC_read_ind_core.vi"("base"=w445) -> ("addr"=w444:u16)  [unwired: 10 in]
      n314 = call "CPU_MEM_read_mem.vi"("address"=w444) -> ("value out"=w443:u8)  [unwired: 10 in]
      n315 = Exclusive Or(1:w443, 2:w452) -> (0:w449:u8)
      n316 = Bundle By Name(cluster=w454, "A"=w449) -> (w451:T1)
      n317 = call "CPU_P_update_ZN.vi"("value"=w449, "registers"=w451) -> ("registers"=w450:T1)  [unwired: 9 in]
    }
    frame 69 {
      # "EOR zp"
      n318 = Unbundle By Name(w462) -> ("PC"=w463:u16, "A"=w461:u8)
      n319 = call "CPU_PC_inc.vi"("registers"=w462) -> ("registers"=w464:T1)  [unwired: 10 in]
      n320 = call "CPU_MEM_read_mem.vi"("address"=w463) -> ("value out"=w456:u8)  [unwired: 10 in]
      n321 = To Unsigned Word Integer(number=w456) -> (unsigned 16bit integer=w455:u16)
      n322 = call "CPU_MEM_read_mem.vi"("address"=w455) -> ("value out"=w457:u8)  [unwired: 10 in]
      n323 = Exclusive Or(1:w457, 2:w461) -> (0:w458:u8)
      n324 = Bundle By Name(cluster=w464, "A"=w458) -> (w460:T1)
      n325 = call "CPU_P_update_ZN.vi"("value"=w458, "registers"=w460) -> ("registers"=w459:T1)  [unwired: 9 in]
    }
    frame 70 {
      # "dx"
      # "LSR zp"
      n326 = Unbundle By Name(w468) -> ("PC"=w470:u16)
      n327 = call "CPU_MEM_read_mem.vi"("address"=w470) -> ("value out"=w469:u8)  [unwired: 10 in]
      n328 = To Unsigned Word Integer(number=w469) -> (unsigned 16bit integer=w466:u16)
      n329 = call "CPU_MEM_read_mem.vi"("address"=w466) -> ("value out"=w467:u8)  [unwired: 10 in]
      n330 = And(x=w467, y=u8 1 ("base")) -> (x .and. y?=w475:u8)
      n331 = Not Equal To 0?(x=w475) -> (x != 0?=w474:bool)
      n332 = call "CPU_P_update.vi"("flag"=enum8{"C", "Z", "I", "D", "B", "V", "N"}."C", "Value"=w474, "registers"=w468) -> ("registers"=w472:T1)  [unwired: 8 in]
      n333 = Logical Shift(y=i16 -1, x=w467) -> (x << y=w465:u8)
      n334 = call "CPU_P_update_ZN.vi"("value"=w465, "registers"=w472) -> ("registers"=w471:T1)  [unwired: 9 in]
      n335 = call "CPU_MEM_write_mem.vi"("value"=w465, "address"=w466) -> ()  [unwired: 10 in]
      n336 = call "CPU_PC_inc.vi"("registers"=w471) -> ("registers"=w478:T1)  [unwired: 10 in]
    }
    frame 72 {
      # "PHA"
      n337 = Unbundle By Name(w480) -> ("A"=w481:u8)
      n338 = call "CPU_SP_push.vi"("value"=w481, "registers"=w480) -> ("registers"=w479:T1)  [unwired: 9 in]
    }
    frame 73 {
      # "EOR imm"
      n339 = Unbundle By Name(w482) -> ("PC"=w489:u16, "A"=w488:u8)
      n340 = call "CPU_PC_inc.vi"("registers"=w482) -> ("registers"=w483:T1)  [unwired: 10 in]
      n341 = call "CPU_MEM_read_mem.vi"("address"=w489) -> ("value out"=w487:u8)  [unwired: 10 in]
      n342 = Exclusive Or(1:w487, 2:w488) -> (0:w484:u8)
      n343 = Bundle By Name(cluster=w483, "A"=w484) -> (w486:T1)
      n344 = call "CPU_P_update_ZN.vi"("value"=w484, "registers"=w486) -> ("registers"=w485:T1)  [unwired: 9 in]
    }
    frame 74 {
      # "dx"
      # "LSR A"
      n345 = Unbundle By Name(w499) -> ("A"=w495:u8)
      n346 = And(x=w495, y=u8 1 ("base")) -> (x .and. y?=w497:u8)
      n347 = Not Equal To 0?(x=w497) -> (x != 0?=w496:bool)
      n348 = Logical Shift(y=i16 -1, x=w495) -> (x << y=w490:u8)
      n349 = call "CPU_P_update.vi"("flag"=enum8{"C", "Z", "I", "D", "B", "V", "N"}."C", "Value"=w496, "registers"=w499) -> ("registers"=w492:T1)  [unwired: 8 in]
      n350 = Bundle By Name(cluster=w492, "A"=w490) -> (w491:T1)
      n351 = call "CPU_P_update_ZN.vi"("value"=w490, "registers"=w491) -> ("registers"=w493:T1)  [unwired: 9 in]
    }
    frame 76 {
      # "JMP abs"
      n352 = call "CPU_MEM_read_mem_16.vi"("registers"=w503) -> ("value"=w501:u16, "registers"=w502:T1)  [unwired: 9 in]
      n353 = Bundle By Name(cluster=w502, "PC"=w501) -> (w504:T1)
    }
    frame 77 {
      # "EOR abs"
      n354 = Unbundle By Name(w507) -> ("A"=w512:u8)
      n355 = call "CPU_MEM_read_mem_16.vi"("registers"=w507) -> ("value"=w505:u16, "registers"=w506:T1)  [unwired: 9 in]
      n356 = call "CPU_MEM_read_mem.vi"("address"=w505) -> ("value out"=w508:u8)  [unwired: 10 in]
      n357 = Exclusive Or(1:w508, 2:w512) -> (0:w509:u8)
      n358 = Bundle By Name(cluster=w506, "A"=w509) -> (w511:T1)
      n359 = call "CPU_P_update_ZN.vi"("value"=w509, "registers"=w511) -> ("registers"=w510:T1)  [unwired: 9 in]
    }
    frame 78 {
      # "dx"
      # "LSR abs"
      n360 = call "CPU_MEM_read_mem_16.vi"("registers"=w515) -> ("value"=w513:u16, "registers"=w514:T1)  [unwired: 9 in]
      n361 = call "CPU_MEM_read_mem.vi"("address"=w513) -> ("value out"=w518:u8)  [unwired: 10 in]
      n362 = And(x=w518, y=u8 1 ("base")) -> (x .and. y?=w522:u8)
      n363 = Not Equal To 0?(x=w522) -> (x != 0?=w521:bool)
      n364 = Logical Shift(y=i16 -1, x=w518) -> (x << y=w516:u8)
      n365 = call "CPU_P_update.vi"("flag"=enum8{"C", "Z", "I", "D", "B", "V", "N"}."C", "Value"=w521, "registers"=w514) -> ("registers"=w517:T1)  [unwired: 8 in]
      n366 = call "CPU_MEM_write_mem.vi"("value"=w516, "address"=w513) -> ()  [unwired: 10 in]
      n367 = call "CPU_P_update_ZN.vi"("value"=w516, "registers"=w517) -> ("registers"=w519:T1)  [unwired: 9 in]
    }
    frame 80 {
      # "BVC"
      n368 = call "OC_Branch_core.vi"("if set/clear"=FALSE, "flag"=enum8{"C", "Z", "I", "D", "B", "V", "N"}."V", "registers"=w526) -> ("registers"=w525:T1)  [unwired: 8 in]
    }
    frame 81 {
      # "EOR indy"
      n369 = Unbundle By Name(w539) -> ("PC"=w534:u16, "A"=w538:u8, "Y"=w530:u8)
      n370 = call "CPU_PC_inc.vi"("registers"=w539) -> ("registers"=w540:T1)  [unwired: 10 in]
      n371 = call "CPU_MEM_read_mem.vi"("address"=w534) -> ("value out"=w532:u8)  [unwired: 10 in]
      n372 = call "OC_read_ind_core.vi"("base"=w532) -> ("addr"=w531:u16)  [unwired: 10 in]
      n373 = Add(x=w531, y=w530) -> (x+y=w529:u16)
      n374 = call "CPU_MEM_read_mem.vi"("address"=w529) -> ("value out"=w533:u8)  [unwired: 10 in]
      n375 = Exclusive Or(1:w533, 2:w538) -> (0:w535:u8)
      n376 = Bundle By Name(cluster=w540, "A"=w535) -> (w537:T1)
      n377 = call "CPU_P_update_ZN.vi"("value"=w535, "registers"=w537) -> ("registers"=w536:T1)  [unwired: 9 in]
    }
    frame 85 {
      # "EOR zpx"
      n378 = Unbundle By Name(w550) -> ("PC"=w551:u16, "A"=w549:u8, "X"=w544:u8)
      n379 = call "CPU_PC_inc.vi"("registers"=w550) -> ("registers"=w552:T1)  [unwired: 10 in]
      n380 = call "CPU_MEM_read_mem.vi"("address"=w551) -> ("value out"=w542:u8)  [unwired: 10 in]
      n381 = Add(x=w542, y=w544) -> (x+y=w543:u8)
      n382 = To Unsigned Word Integer(number=w543) -> (unsigned 16bit integer=w541:u16)
      n383 = call "CPU_MEM_read_mem.vi"("address"=w541) -> ("value out"=w545:u8)  [unwired: 10 in]
      n384 = Exclusive Or(1:w545, 2:w549) -> (0:w546:u8)
      n385 = Bundle By Name(cluster=w552, "A"=w546) -> (w548:T1)
      n386 = call "CPU_P_update_ZN.vi"("value"=w546, "registers"=w548) -> ("registers"=w547:T1)  [unwired: 9 in]
    }
    frame 86 {
      # "dx"
      # "LSR zp X"
      n387 = Unbundle By Name(w559) -> ("PC"=w560:u16, "X"=w555:u8)
      n388 = call "CPU_MEM_read_mem.vi"("address"=w560) -> ("value out"=w554:u8)  [unwired: 10 in]
      n389 = Add(x=w554, y=w555) -> (x+y=w553:u8)
      n390 = To Unsigned Word Integer(number=w553) -> (unsigned 16bit integer=w557:u16)
      n391 = call "CPU_MEM_read_mem.vi"("address"=w557) -> ("value out"=w558:u8)  [unwired: 10 in]
      n392 = And(x=w558, y=u8 1 ("base")) -> (x .and. y?=w565:u8)
      n393 = Logical Shift(y=i16 -1, x=w558) -> (x << y=w556:u8)
      n394 = Not Equal To 0?(x=w565) -> (x != 0?=w564:bool)
      n395 = call "CPU_P_update.vi"("flag"=enum8{"C", "Z", "I", "D", "B", "V", "N"}."C", "Value"=w564, "registers"=w559) -> ("registers"=w562:T1)  [unwired: 8 in]
      n396 = call "CPU_MEM_write_mem.vi"("value"=w556, "address"=w557) -> ()  [unwired: 10 in]
      n397 = call "CPU_P_update_ZN.vi"("value"=w556, "registers"=w562) -> ("registers"=w561:T1)  [unwired: 9 in]
      n398 = call "CPU_PC_inc.vi"("registers"=w561) -> ("registers"=w568:T1)  [unwired: 10 in]
    }
    frame 88 {
      # "CLI"
      n399 = call "CPU_P_update.vi"("flag"=enum8{"C", "Z", "I", "D", "B", "V", "N"}."I", "Value"=FALSE, "registers"=w572) -> ("registers"=w569:T1)  [unwired: 8 in]
    }
    frame 93 {
      # "EOR absx"
      n400 = Unbundle By Name(w575) -> ("A"=w582:u8, "X"=w576:u8)
      n401 = call "CPU_MEM_read_mem_16.vi"("registers"=w575) -> ("value"=w573:u16, "registers"=w574:T1)  [unwired: 9 in]
      n402 = Add(x=w573, y=w576) -> (x+y=w577:u16)
      n403 = call "CPU_MEM_read_mem.vi"("address"=w577) -> ("value out"=w578:u8)  [unwired: 10 in]
      n404 = Exclusive Or(1:w578, 2:w582) -> (0:w579:u8)
      n405 = Bundle By Name(cluster=w574, "A"=w579) -> (w581:T1)
      n406 = call "CPU_P_update_ZN.vi"("value"=w579, "registers"=w581) -> ("registers"=w580:T1)  [unwired: 9 in]
    }
    frame 89 {
      # "EOR absy"
      n407 = Unbundle By Name(w585) -> ("A"=w592:u8, "Y"=w586:u8)
      n408 = call "CPU_MEM_read_mem_16.vi"("registers"=w585) -> ("value"=w583:u16, "registers"=w584:T1)  [unwired: 9 in]
      n409 = Add(x=w583, y=w586) -> (x+y=w587:u16)
      n410 = call "CPU_MEM_read_mem.vi"("address"=w587) -> ("value out"=w588:u8)  [unwired: 10 in]
      n411 = Exclusive Or(1:w588, 2:w592) -> (0:w589:u8)
      n412 = Bundle By Name(cluster=w584, "A"=w589) -> (w591:T1)
      n413 = call "CPU_P_update_ZN.vi"("value"=w589, "registers"=w591) -> ("registers"=w590:T1)  [unwired: 9 in]
    }
    frame 94 {
      # "dx"
      # "LSR abs X"
      n414 = Unbundle By Name(w595) -> ("X"=w596:u8)
      n415 = call "CPU_MEM_read_mem_16.vi"("registers"=w595) -> ("value"=w593:u16, "registers"=w594:T1)  [unwired: 9 in]
      n416 = Add(x=w593, y=w596) -> (x+y=w597:u16)
      n417 = call "CPU_MEM_read_mem.vi"("address"=w597) -> ("value out"=w600:u8)  [unwired: 10 in]
      n418 = And(x=w600, y=u8 1 ("base")) -> (x .and. y?=w604:u8)
      n419 = Logical Shift(y=i16 -1, x=w600) -> (x << y=w598:u8)
      n420 = Not Equal To 0?(x=w604) -> (x != 0?=w603:bool)
      n421 = call "CPU_P_update.vi"("flag"=enum8{"C", "Z", "I", "D", "B", "V", "N"}."C", "Value"=w603, "registers"=w594) -> ("registers"=w599:T1)  [unwired: 8 in]
      n422 = call "CPU_MEM_write_mem.vi"("value"=w598, "address"=w597) -> ()  [unwired: 10 in]
      n423 = call "CPU_P_update_ZN.vi"("value"=w598, "registers"=w599) -> ("registers"=w601:T1)  [unwired: 9 in]
    }
    frame 96 {
      # "RTS"
      n424 = Unbundle By Name(w610) -> ("SP"=w619:u8)
      n425 = Increment(x=w619) -> (x+1=w614:u8)
      n426 = Add(x=w614, y=u16 256) -> (x+y=w617:u16)
      n427 = call "CPU_MEM_read_mem.vi"("address"=w617) -> ("value out"=w613:u8)  [unwired: 10 in]
      n428 = Increment(x=w614) -> (x+1=w608:u8)
      n429 = Add(x=w608, y=u16 256) -> (x+y=w616:u16)
      n430 = call "CPU_MEM_read_mem.vi"("address"=w616) -> ("value out"=w612:u8)  [unwired: 10 in]
      n431 = Join Numbers(hi=w612, lo=w613) -> ((hi.lo)=w611:u16)
      n432 = Increment(x=w611) -> (x+1=w607:u16)
      n433 = Bundle By Name(cluster=w610, "SP"=w608, "PC"=w607) -> (w609:T1)
    }
    frame 97 {
      # "ADC indx"
      n434 = Unbundle By Name(w628) -> ("PC"=w626:u16, "X"=w627:u8)
      n435 = call "CPU_PC_inc.vi"("registers"=w628) -> ("registers"=w622:T1)  [unwired: 10 in]
      n436 = call "CPU_MEM_read_mem.vi"("address"=w626) -> ("value out"=w625:u8)  [unwired: 10 in]
      n437 = Add(x=w625, y=w627) -> (x+y=w624:u8)
      n438 = call "OC_read_ind_core.vi"("base"=w624) -> ("addr"=w623:u16)  [unwired: 10 in]
      n439 = call "CPU_MEM_read_mem.vi"("address"=w623) -> ("value out"=w620:u8)  [unwired: 10 in]
      n440 = call "OC_ADC_core.vi"("value"=w620, "registers"=w622) -> ("registers"=w621:T1)  [unwired: 9 in]
    }
    frame 101 {
      # "ADC zp"
      # "ADC"
      n441 = Unbundle By Name(w634) -> ("PC"=w635:u16)
      n442 = call "CPU_PC_inc.vi"("registers"=w634) -> ("registers"=w633:T1)  [unwired: 10 in]
      n443 = call "CPU_MEM_read_mem.vi"("address"=w635) -> ("value out"=w631:u8)  [unwired: 10 in]
      n444 = To Unsigned Word Integer(number=w631) -> (unsigned 16bit integer=w629:u16)
      n445 = call "CPU_MEM_read_mem.vi"("address"=w629) -> ("value out"=w630:u8)  [unwired: 10 in]
      n446 = call "OC_ADC_core.vi"("value"=w630, "registers"=w633) -> ("registers"=w632:T1)  [unwired: 9 in]
    }
    frame 117 {
      # "ADC zp X"
      # "ADC"
      n447 = Unbundle By Name(w643) -> ("PC"=w644:u16, "X"=w636:u8)
      n448 = call "CPU_PC_inc.vi"("registers"=w643) -> ("registers"=w642:T1)  [unwired: 10 in]
      n449 = call "CPU_MEM_read_mem.vi"("address"=w644) -> ("value out"=w640:u8)  [unwired: 10 in]
      n450 = Add(x=w640, y=w636) -> (x+y=w637:u8)
      n451 = To Unsigned Word Integer(number=w637) -> (unsigned 16bit integer=w638:u16)
      n452 = call "CPU_MEM_read_mem.vi"("address"=w638) -> ("value out"=w639:u8)  [unwired: 10 in]
      n453 = call "OC_ADC_core.vi"("value"=w639, "registers"=w642) -> ("registers"=w641:T1)  [unwired: 9 in]
    }
    frame 102 {
      # "dx"
      # "ROR zp"
      n454 = Unbundle By Name(w647) -> ("PC"=w659:u16)
      n455 = call "CPU_MEM_read_mem.vi"("address"=w659) -> ("value out"=w658:u8)  [unwired: 10 in]
      n456 = To Unsigned Word Integer(number=w658) -> (unsigned 16bit integer=w649:u16)
      n457 = call "CPU_P_get_flag.vi"("flag"=enum8{"C", "Z", "I", "D", "B", "V", "N"}."C", "registers"=w647) -> ("Value"=w655:bool)  [unwired: 8 in, 1 out]
      n458 = call "CPU_MEM_read_mem.vi"("address"=w649) -> ("value out"=w657:u8)  [unwired: 10 in]
      n459 = Boolean To (0,1)(Boolean=w655) -> (0, 1=w654:i16)
      n460 = To Unsigned Byte Integer(number=w654) -> (unsigned 8bit integer=w653:u8)
      n461 = And(x=w657, y=u8 1 ("base")) -> (x .and. y?=w662:u8)
      n462 = Logical Shift(y=i16 -1, x=w657) -> (x << y=w650:u8)
      n463 = Logical Shift(y=i16 7, x=w653) -> (x << y=w651:u8)
      n464 = Not Equal To 0?(x=w662) -> (x != 0?=w661:bool)
      n465 = Or(x=w650, y=w651) -> (x .or. y?=w648:u8)
      n466 = call "CPU_P_update_ZN.vi"("value"=w648, "registers"=w647) -> ("registers"=w646:T1)  [unwired: 9 in]
      n467 = call "CPU_MEM_write_mem.vi"("value"=w648, "address"=w649) -> ()  [unwired: 10 in]
      n468 = call "CPU_P_update.vi"("flag"=enum8{"C", "Z", "I", "D", "B", "V", "N"}."C", "Value"=w661, "registers"=w646) -> ("registers"=w645:T1)  [unwired: 8 in]
      n469 = call "CPU_PC_inc.vi"("registers"=w645) -> ("registers"=w665:T1)  [unwired: 10 in]
    }
    frame 104 {
      # "PLA"
      n470 = call "CPU_SP_pop.vi"("registers"=w668) -> ("value"=w667:u8, "registers"=w666:T1)  [unwired: 9 in]
      n471 = Bundle By Name(cluster=w666, "A"=w667) -> (w670:T1)
      n472 = call "CPU_P_update_ZN.vi"("value"=w667, "registers"=w670) -> ("registers"=w669:T1)  [unwired: 9 in]
    }
    frame 105 {
      # "ADC imm"
      # "ADC"
      n473 = Unbundle By Name(w674) -> ("PC"=w675:u16)
      n474 = call "CPU_PC_inc.vi"("registers"=w674) -> ("registers"=w673:T1)  [unwired: 10 in]
      n475 = call "CPU_MEM_read_mem.vi"("address"=w675) -> ("value out"=w671:u8)  [unwired: 10 in]
      n476 = call "OC_ADC_core.vi"("value"=w671, "registers"=w673) -> ("registers"=w672:T1)  [unwired: 9 in]
    }
    frame 106 {
      # "dx"
      # "ROR A"
      n477 = call "CPU_P_get_flag.vi"("flag"=enum8{"C", "Z", "I", "D", "B", "V", "N"}."C", "registers"=w677) -> ("Value"=w685:bool)  [unwired: 8 in, 1 out]
      n478 = Unbundle By Name(w677) -> ("A"=w689:u8)
      n479 = Boolean To (0,1)(Boolean=w685) -> (0, 1=w684:i16)
      n480 = To Unsigned Byte Integer(number=w684) -> (unsigned 8bit integer=w683:u8)
      n481 = And(x=w689, y=u8 1 ("base")) -> (x .and. y?=w691:u8)
      n482 = Logical Shift(y=i16 -1, x=w689) -> (x << y=w687:u8)
      n483 = Not Equal To 0?(x=w691) -> (x != 0?=w690:bool)
      n484 = Logical Shift(y=i16 7, x=w683) -> (x << y=w681:u8)
      n485 = Or(x=w687, y=w681) -> (x .or. y?=w679:u8)
      n486 = Bundle By Name(cluster=w677, "A"=w679) -> (w678:T1)
      n487 = call "CPU_P_update.vi"("flag"=enum8{"C", "Z", "I", "D", "B", "V", "N"}."C", "Value"=w690, "registers"=w678) -> ("registers"=w676:T1)  [unwired: 8 in]
      n488 = call "CPU_P_update_ZN.vi"("value"=w679, "registers"=w676) -> ("registers"=w680:T1)  [unwired: 9 in]
    }
    frame 108 {
      # "Attenzione: il 6502 ha un bug se ptr è a fine pagina (xxFF)"
      # "JMP ind"
      # "ADC"
      n489 = call "CPU_MEM_read_mem_16.vi"("registers"=w696) -> ("value"=w694:u16, "registers"=w695:T1)  [unwired: 9 in]
      n490 = Increment(x=w694) -> (x+1=w697:u16)
      n491 = call "CPU_MEM_read_mem.vi"("address"=w694) -> ("value out"=w700:u8)  [unwired: 10 in]
      n492 = call "CPU_MEM_read_mem.vi"("address"=w697) -> ("value out"=w701:u8)  [unwired: 10 in]
      n493 = Join Numbers(hi=w701, lo=w700) -> ((hi.lo)=w698:u16)
      n494 = Bundle By Name(cluster=w695, "PC"=w698) -> (w699:T1)
    }
    frame 109 {
      # "ADC abs"
      # "ADC"
      n495 = call "CPU_MEM_read_mem_16.vi"("registers"=w704) -> ("value"=w703:u16, "registers"=w702:T1)  [unwired: 9 in]
      n496 = call "CPU_MEM_read_mem.vi"("address"=w703) -> ("value out"=w705:u8)  [unwired: 10 in]
      n497 = call "OC_ADC_core.vi"("value"=w705, "registers"=w702) -> ("registers"=w706:T1)  [unwired: 9 in]
    }
    frame 125 {
      # "ADC abs X"
      # "ADC"
      n498 = Unbundle By Name(w709) -> ("X"=w710:u8)
      n499 = call "CPU_MEM_read_mem_16.vi"("registers"=w709) -> ("value"=w707:u16, "registers"=w708:T1)  [unwired: 9 in]
      n500 = Add(x=w707, y=w710) -> (x+y=w711:u16)
      n501 = call "CPU_MEM_read_mem.vi"("address"=w711) -> ("value out"=w712:u8)  [unwired: 10 in]
      n502 = call "OC_ADC_core.vi"("value"=w712, "registers"=w708) -> ("registers"=w713:T1)  [unwired: 9 in]
    }
    frame 121 {
      # "ADC abs Y"
      # "ADC"
      n503 = Unbundle By Name(w716) -> ("Y"=w717:u8)
      n504 = call "CPU_MEM_read_mem_16.vi"("registers"=w716) -> ("value"=w714:u16, "registers"=w715:T1)  [unwired: 9 in]
      n505 = Add(x=w714, y=w717) -> (x+y=w718:u16)
      n506 = call "CPU_MEM_read_mem.vi"("address"=w718) -> ("value out"=w719:u8)  [unwired: 10 in]
      n507 = call "OC_ADC_core.vi"("value"=w719, "registers"=w715) -> ("registers"=w720:T1)  [unwired: 9 in]
    }
    frame 110 {
      # "dx"
      # "ROR abs"
      n508 = call "CPU_MEM_read_mem_16.vi"("registers"=w723) -> ("value"=w721:u16, "registers"=w722:T1)  [unwired: 9 in]
      n509 = call "CPU_MEM_read_mem.vi"("address"=w721) -> ("value out"=w728:u8)  [unwired: 10 in]
      n510 = call "CPU_P_get_flag.vi"("flag"=enum8{"C", "Z", "I", "D", "B", "V", "N"}."C", "registers"=w723) -> ("Value"=w733:bool)  [unwired: 8 in, 1 out]
      n511 = Boolean To (0,1)(Boolean=w733) -> (0, 1=w732:i16)
      n512 = To Unsigned Byte Integer(number=w732) -> (unsigned 8bit integer=w725:u8)
      n513 = And(x=w728, y=u8 1 ("base")) -> (x .and. y?=w737:u8)
      n514 = Logical Shift(y=i16 -1, x=w728) -> (x << y=w731:u8)
      n515 = Logical Shift(y=i16 7, x=w725) -> (x << y=w724:u8)
      n516 = Not Equal To 0?(x=w737) -> (x != 0?=w736:bool)
      n517 = Or(x=w731, y=w724) -> (x .or. y?=w730:u8)
      n518 = call "CPU_MEM_write_mem.vi"("value"=w730, "address"=w721) -> ()  [unwired: 10 in]
      n519 = call "CPU_P_update_ZN.vi"("value"=w730, "registers"=w722) -> ("registers"=w729:T1)  [unwired: 9 in]
      n520 = call "CPU_P_update.vi"("flag"=enum8{"C", "Z", "I", "D", "B", "V", "N"}."C", "Value"=w736, "registers"=w729) -> ("registers"=w727:T1)  [unwired: 8 in]
    }
    frame 112 {
      # "BVS"
      n521 = call "OC_Branch_core.vi"("if set/clear"=TRUE, "flag"=enum8{"C", "Z", "I", "D", "B", "V", "N"}."V", "registers"=w741) -> ("registers"=w740:T1)  [unwired: 8 in]
    }
    frame 113 {
      # "ADC indy"
      n522 = Unbundle By Name(w752) -> ("PC"=w751:u16, "Y"=w746:u8)
      n523 = call "CPU_PC_inc.vi"("registers"=w752) -> ("registers"=w750:T1)  [unwired: 10 in]
      n524 = call "CPU_MEM_read_mem.vi"("address"=w751) -> ("value out"=w747:u8)  [unwired: 10 in]
      n525 = call "OC_read_ind_core.vi"("base"=w747) -> ("addr"=w745:u16)  [unwired: 10 in]
      n526 = Add(x=w745, y=w746) -> (x+y=w744:u16)
      n527 = call "CPU_MEM_read_mem.vi"("address"=w744) -> ("value out"=w748:u8)  [unwired: 10 in]
      n528 = call "OC_ADC_core.vi"("value"=w748, "registers"=w750) -> ("registers"=w749:T1)  [unwired: 9 in]
    }
    frame 118 {
      # "dx"
      # "ROR zp"
      n529 = Unbundle By Name(w758) -> ("PC"=w769:u16, "X"=w755:u8)
      n530 = call "CPU_MEM_read_mem.vi"("address"=w769) -> ("value out"=w754:u8)  [unwired: 10 in]
      n531 = Add(x=w754, y=w755) -> (x+y=w753:u8)
      n532 = call "CPU_P_get_flag.vi"("flag"=enum8{"C", "Z", "I", "D", "B", "V", "N"}."C", "registers"=w758) -> ("Value"=w766:bool)  [unwired: 8 in, 1 out]
      n533 = To Unsigned Word Integer(number=w753) -> (unsigned 16bit integer=w760:u16)
      n534 = Boolean To (0,1)(Boolean=w766) -> (0, 1=w765:i16)
      n535 = call "CPU_MEM_read_mem.vi"("address"=w760) -> ("value out"=w768:u8)  [unwired: 10 in]
      n536 = To Unsigned Byte Integer(number=w765) -> (unsigned 8bit integer=w764:u8)
      n537 = And(x=w768, y=u8 1 ("base")) -> (x .and. y?=w772:u8)
      n538 = Logical Shift(y=i16 7, x=w764) -> (x << y=w762:u8)
      n539 = Logical Shift(y=i16 -1, x=w768) -> (x << y=w761:u8)
      n540 = Not Equal To 0?(x=w772) -> (x != 0?=w771:bool)
      n541 = Or(x=w761, y=w762) -> (x .or. y?=w759:u8)
      n542 = call "CPU_P_update_ZN.vi"("value"=w759, "registers"=w758) -> ("registers"=w757:T1)  [unwired: 9 in]
      n543 = call "CPU_MEM_write_mem.vi"("value"=w759, "address"=w760) -> ()  [unwired: 10 in]
      n544 = call "CPU_P_update.vi"("flag"=enum8{"C", "Z", "I", "D", "B", "V", "N"}."C", "Value"=w771, "registers"=w757) -> ("registers"=w756:T1)  [unwired: 8 in]
      n545 = call "CPU_PC_inc.vi"("registers"=w756) -> ("registers"=w775:T1)  [unwired: 10 in]
    }
    frame 120 {
      # "SEI"
      n546 = call "CPU_P_update.vi"("flag"=enum8{"C", "Z", "I", "D", "B", "V", "N"}."I", "Value"=TRUE, "registers"=w779) -> ("registers"=w776:T1)  [unwired: 8 in]
    }
    frame 126 {
      # "dx"
      # "ROR abs X"
      n547 = call "CPU_MEM_read_mem_16.vi"("registers"=w782) -> ("value"=w780:u16, "registers"=w781:T1)  [unwired: 9 in]
      n548 = Unbundle By Name(w782) -> ("X"=w783:u8)
      n549 = Add(x=w780, y=w783) -> (x+y=w784:u16)
      n550 = call "CPU_MEM_read_mem.vi"("address"=w784) -> ("value out"=w789:u8)  [unwired: 10 in]
      n551 = call "CPU_P_get_flag.vi"("flag"=enum8{"C", "Z", "I", "D", "B", "V", "N"}."C", "registers"=w782) -> ("Value"=w794:bool)  [unwired: 8 in, 1 out]
      n552 = Boolean To (0,1)(Boolean=w794) -> (0, 1=w793:i16)
      n553 = To Unsigned Byte Integer(number=w793) -> (unsigned 8bit integer=w786:u8)
      n554 = And(x=w789, y=u8 1 ("base")) -> (x .and. y?=w798:u8)
      n555 = Logical Shift(y=i16 -1, x=w789) -> (x << y=w792:u8)
      n556 = Logical Shift(y=i16 7, x=w786) -> (x << y=w785:u8)
      n557 = Not Equal To 0?(x=w798) -> (x != 0?=w797:bool)
      n558 = Or(x=w792, y=w785) -> (x .or. y?=w791:u8)
      n559 = call "CPU_P_update_ZN.vi"("value"=w791, "registers"=w781) -> ("registers"=w790:T1)  [unwired: 9 in]
      n560 = call "CPU_MEM_write_mem.vi"("value"=w791, "address"=w784) -> ()  [unwired: 10 in]
      n561 = call "CPU_P_update.vi"("flag"=enum8{"C", "Z", "I", "D", "B", "V", "N"}."C", "Value"=w797, "registers"=w790) -> ("registers"=w788:T1)  [unwired: 8 in]
    }
    frame 129 {
      # "STA indx"
      n562 = Unbundle By Name(w808) -> ("PC"=w806:u16, "X"=w807:u8, "A"=w801:u8)
      n563 = call "CPU_PC_inc.vi"("registers"=w808) -> ("registers"=w803:T1)  [unwired: 10 in]
      n564 = call "CPU_MEM_read_mem.vi"("address"=w806) -> ("value out"=w805:u8)  [unwired: 10 in]
      n565 = Add(x=w805, y=w807) -> (x+y=w804:u8)
      n566 = call "OC_read_ind_core.vi"("base"=w804) -> ("addr"=w802:u16)  [unwired: 10 in]
      n567 = call "CPU_MEM_write_mem.vi"("value"=w801, "address"=w802) -> ()  [unwired: 10 in]
    }
    frame 132 {
      # "STY zp"
      n568 = Unbundle By Name(w813) -> ("PC"=w814:u16)
      n569 = call "CPU_PC_inc.vi"("registers"=w813) -> ("registers"=w811:T1)  [unwired: 10 in]
      n570 = call "CPU_MEM_read_mem.vi"("address"=w814) -> ("value out"=w810:u8)  [unwired: 10 in]
      n571 = To Unsigned Word Integer(number=w810) -> (unsigned 16bit integer=w809:u16)
      n572 = Unbundle By Name(w811) -> ("Y"=w812:u8)
      n573 = call "CPU_MEM_write_mem.vi"("value"=w812, "address"=w809) -> ()  [unwired: 10 in]
    }
    frame 133 {
      # "STA zp"
      n574 = Unbundle By Name(w819) -> ("PC"=w820:u16)
      n575 = call "CPU_PC_inc.vi"("registers"=w819) -> ("registers"=w817:T1)  [unwired: 10 in]
      n576 = call "CPU_MEM_read_mem.vi"("address"=w820) -> ("value out"=w816:u8)  [unwired: 10 in]
      n577 = To Unsigned Word Integer(number=w816) -> (unsigned 16bit integer=w815:u16)
      n578 = Unbundle By Name(w817) -> ("A"=w818:u8)
      n579 = call "CPU_MEM_write_mem.vi"("value"=w818, "address"=w815) -> ()  [unwired: 10 in]
    }
    frame 134 {
      # "STX zp"
      n580 = Unbundle By Name(w825) -> ("PC"=w826:u16)
      n581 = call "CPU_PC_inc.vi"("registers"=w825) -> ("registers"=w823:T1)  [unwired: 10 in]
      n582 = call "CPU_MEM_read_mem.vi"("address"=w826) -> ("value out"=w822:u8)  [unwired: 10 in]
      n583 = To Unsigned Word Integer(number=w822) -> (unsigned 16bit integer=w821:u16)
      n584 = Unbundle By Name(w823) -> ("X"=w824:u8)
      n585 = call "CPU_MEM_write_mem.vi"("value"=w824, "address"=w821) -> ()  [unwired: 10 in]
    }
    frame 136 {
      # "DEY"
      n586 = Unbundle By Name(w831) -> ("Y"=w829:u8)
      n587 = Decrement(x=w829) -> (x-1=w828:u8)
      n588 = Bundle By Name(cluster=w831, "Y"=w828) -> (w830:T1)
      n589 = call "CPU_P_update_ZN.vi"("value"=w828, "registers"=w830) -> ("registers"=w827:T1)  [unwired: 9 in]
    }
    frame 138 {
      # "TXA"
      n590 = Unbundle By Name(w835) -> ("X"=w833:u8)
      n591 = Bundle By Name(cluster=w835, "A"=w833) -> (w834:T1)
      n592 = call "CPU_P_update_ZN.vi"("value"=w833, "registers"=w834) -> ("registers"=w832:T1)  [unwired: 9 in]
    }
    frame 140 {
      # "STY"
      n593 = call "CPU_MEM_read_mem_16.vi"("registers"=w838) -> ("value"=w836:u16, "registers"=w837:T1)  [unwired: 9 in]
      n594 = Unbundle By Name(w837) -> ("Y"=w839:u8)
      n595 = call "CPU_MEM_write_mem.vi"("value"=w839, "address"=w836) -> ()  [unwired: 10 in]
    }
    frame 141 {
      # "STA"
      n596 = call "CPU_MEM_read_mem_16.vi"("registers"=w842) -> ("value"=w840:u16, "registers"=w841:T1)  [unwired: 9 in]
      n597 = Unbundle By Name(w841) -> ("A"=w843:u8)
      n598 = call "CPU_MEM_write_mem.vi"("value"=w843, "address"=w840) -> ()  [unwired: 10 in]
    }
    frame 142 {
      # "STX"
      n599 = call "CPU_MEM_read_mem_16.vi"("registers"=w846) -> ("value"=w844:u16, "registers"=w845:T1)  [unwired: 9 in]
      n600 = Unbundle By Name(w845) -> ("X"=w847:u8)
      n601 = call "CPU_MEM_write_mem.vi"("value"=w847, "address"=w844) -> ()  [unwired: 10 in]
    }
    frame 144 {
      # "BCC"
      n602 = call "OC_Branch_core.vi"("if set/clear"=FALSE, "flag"=enum8{"C", "Z", "I", "D", "B", "V", "N"}."C", "registers"=w849) -> ("registers"=w848:T1)  [unwired: 8 in]
    }
    frame 145 {
      # "STA indy"
      n603 = Unbundle By Name(w859) -> ("PC"=w858:u16, "Y"=w856:u8, "A"=w852:u8)
      n604 = call "CPU_PC_inc.vi"("registers"=w859) -> ("registers"=w854:T1)  [unwired: 10 in]
      n605 = call "CPU_MEM_read_mem.vi"("address"=w858) -> ("value out"=w857:u8)  [unwired: 10 in]
      n606 = call "OC_read_ind_core.vi"("base"=w857) -> ("addr"=w855:u16)  [unwired: 10 in]
      n607 = Add(x=w855, y=w856) -> (x+y=w853:u16)
      n608 = call "CPU_MEM_write_mem.vi"("value"=w852, "address"=w853) -> ()  [unwired: 10 in]
    }
    frame 148 {
      # "STY zp X"
      n609 = Unbundle By Name(w866) -> ("PC"=w867:u16, "X"=w863:u8)
      n610 = call "CPU_PC_inc.vi"("registers"=w866) -> ("registers"=w864:T1)  [unwired: 10 in]
      n611 = call "CPU_MEM_read_mem.vi"("address"=w867) -> ("value out"=w862:u8)  [unwired: 10 in]
      n612 = Add(x=w863, y=w862) -> (x+y=w860:u8)
      n613 = To Unsigned Word Integer(number=w860) -> (unsigned 16bit integer=w861:u16)
      n614 = Unbundle By Name(w864) -> ("Y"=w865:u8)
      n615 = call "CPU_MEM_write_mem.vi"("value"=w865, "address"=w861) -> ()  [unwired: 10 in]
    }
    frame 149 {
      # "STA zp X"
      n616 = Unbundle By Name(w874) -> ("PC"=w875:u16, "X"=w870:u8)
      n617 = call "CPU_PC_inc.vi"("registers"=w874) -> ("registers"=w872:T1)  [unwired: 10 in]
      n618 = call "CPU_MEM_read_mem.vi"("address"=w875) -> ("value out"=w869:u8)  [unwired: 10 in]
      n619 = Add(x=w870, y=w869) -> (x+y=w871:u8)
      n620 = To Unsigned Word Integer(number=w871) -> (unsigned 16bit integer=w868:u16)
      n621 = Unbundle By Name(w872) -> ("A"=w873:u8)
      n622 = call "CPU_MEM_write_mem.vi"("value"=w873, "address"=w868) -> ()  [unwired: 10 in]
    }
    frame 150 {
      # "STX addr Y"
      n623 = Unbundle By Name(w882) -> ("PC"=w883:u16, "Y"=w878:u8)
      n624 = call "CPU_PC_inc.vi"("registers"=w882) -> ("registers"=w880:T1)  [unwired: 10 in]
      n625 = call "CPU_MEM_read_mem.vi"("address"=w883) -> ("value out"=w877:u8)  [unwired: 10 in]
      n626 = Add(x=w878, y=w877) -> (x+y=w879:u8)
      n627 = To Unsigned Word Integer(number=w879) -> (unsigned 16bit integer=w876:u16)
      n628 = Unbundle By Name(w880) -> ("X"=w881:u8)
      n629 = call "CPU_MEM_write_mem.vi"("value"=w881, "address"=w876) -> ()  [unwired: 10 in]
    }
    frame 152 {
      # "TYA"
      n630 = Unbundle By Name(w887) -> ("Y"=w885:u8)
      n631 = Bundle By Name(cluster=w887, "A"=w885) -> (w886:T1)
      n632 = call "CPU_P_update_ZN.vi"("value"=w885, "registers"=w886) -> ("registers"=w884:T1)  [unwired: 9 in]
    }
    frame 153 {
      # "STA abs Y"
      n633 = Unbundle By Name(w890) -> ("Y"=w891:u8)
      n634 = call "CPU_MEM_read_mem_16.vi"("registers"=w890) -> ("value"=w888:u16, "registers"=w889:T1)  [unwired: 9 in]
      n635 = Add(x=w888, y=w891) -> (x+y=w892:u16)
      n636 = Unbundle By Name(w889) -> ("A"=w893:u8)
      n637 = call "CPU_MEM_write_mem.vi"("value"=w893, "address"=w892) -> ()  [unwired: 10 in]
    }
    frame 154 {
      # "TXS"
      n638 = Unbundle By Name(w896) -> ("X"=w895:u8)
      n639 = Bundle By Name(cluster=w896, "SP"=w895) -> (w894:T1)
    }
    frame 157 {
      # "STA abs X"
      n640 = Unbundle By Name(w899) -> ("X"=w902:u8)
      n641 = call "CPU_MEM_read_mem_16.vi"("registers"=w899) -> ("value"=w897:u16, "registers"=w898:T1)  [unwired: 9 in]
      n642 = Add(x=w897, y=w902) -> (x+y=w901:u16)
      n643 = Unbundle By Name(w898) -> ("A"=w900:u8)
      n644 = call "CPU_MEM_write_mem.vi"("value"=w900, "address"=w901) -> ()  [unwired: 10 in]
    }
    frame 160 {
      # "LDY imm"
      n645 = Unbundle By Name(w907) -> ("PC"=w908:u16)
      n646 = call "CPU_PC_inc.vi"("registers"=w907) -> ("registers"=w906:T1)  [unwired: 10 in]
      n647 = call "CPU_MEM_read_mem.vi"("address"=w908) -> ("value out"=w903:u8)  [unwired: 10 in]
      n648 = Bundle By Name(cluster=w906, "Y"=w903) -> (w905:T1)
      n649 = call "CPU_P_update_ZN.vi"("value"=w903, "registers"=w905) -> ("registers"=w904:T1)  [unwired: 9 in]
    }
    frame 161 {
      # "LDA ind X"
      n650 = Unbundle By Name(w917) -> ("PC"=w918:u16, "X"=w913:u8)
      n651 = call "CPU_PC_inc.vi"("registers"=w917) -> ("registers"=w912:T1)  [unwired: 10 in]
      n652 = call "CPU_MEM_read_mem.vi"("address"=w918) -> ("value out"=w911:u8)  [unwired: 10 in]
      n653 = Add(x=w911, y=w913) -> (x+y=w910:u8)
      n654 = call "OC_read_ind_core.vi"("base"=w910) -> ("addr"=w909:u16)  [unwired: 10 in]
      n655 = call "CPU_MEM_read_mem.vi"("address"=w909) -> ("value out"=w914:u8)  [unwired: 10 in]
      n656 = Bundle By Name(cluster=w912, "A"=w914) -> (w916:T1)
      n657 = call "CPU_P_update_ZN.vi"("value"=w914, "registers"=w916) -> ("registers"=w915:T1)  [unwired: 9 in]
    }
    frame 162 {
      # "LDX imm"
      n658 = Unbundle By Name(w923) -> ("PC"=w924:u16)
      n659 = call "CPU_PC_inc.vi"("registers"=w923) -> ("registers"=w922:T1)  [unwired: 10 in]
      n660 = call "CPU_MEM_read_mem.vi"("address"=w924) -> ("value out"=w919:u8)  [unwired: 10 in]
      n661 = Bundle By Name(cluster=w922, "X"=w919) -> (w921:T1)
      n662 = call "CPU_P_update_ZN.vi"("value"=w919, "registers"=w921) -> ("registers"=w920:T1)  [unwired: 9 in]
    }
    frame 164 {
      # "LDY zp"
      n663 = Unbundle By Name(w931) -> ("PC"=w932:u16)
      n664 = call "CPU_PC_inc.vi"("registers"=w931) -> ("registers"=w927:T1)  [unwired: 10 in]
      n665 = call "CPU_MEM_read_mem.vi"("address"=w932) -> ("value out"=w926:u8)  [unwired: 10 in]
      n666 = To Unsigned Word Integer(number=w926) -> (unsigned 16bit integer=w925:u16)
      n667 = call "CPU_MEM_read_mem.vi"("address"=w925) -> ("value out"=w928:u8)  [unwired: 10 in]
      n668 = Bundle By Name(cluster=w927, "Y"=w928) -> (w930:T1)
      n669 = call "CPU_P_update_ZN.vi"("value"=w928, "registers"=w930) -> ("registers"=w929:T1)  [unwired: 9 in]
    }
    frame 165 {
      # "LDA zp"
      n670 = Unbundle By Name(w939) -> ("PC"=w940:u16)
      n671 = call "CPU_PC_inc.vi"("registers"=w939) -> ("registers"=w935:T1)  [unwired: 10 in]
      n672 = call "CPU_MEM_read_mem.vi"("address"=w940) -> ("value out"=w934:u8)  [unwired: 10 in]
      n673 = To Unsigned Word Integer(number=w934) -> (unsigned 16bit integer=w933:u16)
      n674 = call "CPU_MEM_read_mem.vi"("address"=w933) -> ("value out"=w936:u8)  [unwired: 10 in]
      n675 = Bundle By Name(cluster=w935, "A"=w936) -> (w938:T1)
      n676 = call "CPU_P_update_ZN.vi"("value"=w936, "registers"=w938) -> ("registers"=w937:T1)  [unwired: 9 in]
    }
    frame 166 {
      # "LDX zp"
      n677 = Unbundle By Name(w947) -> ("PC"=w948:u16)
      n678 = call "CPU_PC_inc.vi"("registers"=w947) -> ("registers"=w943:T1)  [unwired: 10 in]
      n679 = call "CPU_MEM_read_mem.vi"("address"=w948) -> ("value out"=w942:u8)  [unwired: 10 in]
      n680 = To Unsigned Word Integer(number=w942) -> (unsigned 16bit integer=w941:u16)
      n681 = call "CPU_MEM_read_mem.vi"("address"=w941) -> ("value out"=w944:u8)  [unwired: 10 in]
      n682 = Bundle By Name(cluster=w943, "X"=w944) -> (w946:T1)
      n683 = call "CPU_P_update_ZN.vi"("value"=w944, "registers"=w946) -> ("registers"=w945:T1)  [unwired: 9 in]
    }
    frame 168 {
      # "TAY"
      n684 = Unbundle By Name(w952) -> ("A"=w950:u8)
      n685 = Bundle By Name(cluster=w952, "Y"=w950) -> (w951:T1)
      n686 = call "CPU_P_update_ZN.vi"("value"=w950, "registers"=w951) -> ("registers"=w949:T1)  [unwired: 9 in]
    }
    frame 169 {
      # "LDA imm"
      n687 = Unbundle By Name(w957) -> ("PC"=w958:u16)
      n688 = call "CPU_PC_inc.vi"("registers"=w957) -> ("registers"=w956:T1)  [unwired: 10 in]
      n689 = call "CPU_MEM_read_mem.vi"("address"=w958) -> ("value out"=w953:u8)  [unwired: 10 in]
      n690 = Bundle By Name(cluster=w956, "A"=w953) -> (w955:T1)
      n691 = call "CPU_P_update_ZN.vi"("value"=w953, "registers"=w955) -> ("registers"=w954:T1)  [unwired: 9 in]
    }
    frame 170 {
      # "TAX"
      n692 = Unbundle By Name(w962) -> ("A"=w960:u8)
      n693 = Bundle By Name(cluster=w962, "X"=w960) -> (w961:T1)
      n694 = call "CPU_P_update_ZN.vi"("value"=w960, "registers"=w961) -> ("registers"=w959:T1)  [unwired: 9 in]
    }
    frame 172 {
      # "LDY abs"
      n695 = call "CPU_MEM_read_mem_16.vi"("registers"=w965) -> ("value"=w963:u16, "registers"=w964:T1)  [unwired: 9 in]
      n696 = call "CPU_MEM_read_mem.vi"("address"=w963) -> ("value out"=w966:u8)  [unwired: 10 in]
      n697 = Bundle By Name(cluster=w964, "Y"=w966) -> (w968:T1)
      n698 = call "CPU_P_update_ZN.vi"("value"=w966, "registers"=w968) -> ("registers"=w967:T1)  [unwired: 9 in]
    }
    frame 173 {
      # "LDA abs"
      n699 = call "CPU_MEM_read_mem_16.vi"("registers"=w971) -> ("value"=w969:u16, "registers"=w970:T1)  [unwired: 9 in]
      n700 = call "CPU_MEM_read_mem.vi"("address"=w969) -> ("value out"=w972:u8)  [unwired: 10 in]
      n701 = Bundle By Name(cluster=w970, "A"=w972) -> (w974:T1)
      n702 = call "CPU_P_update_ZN.vi"("value"=w972, "registers"=w974) -> ("registers"=w973:T1)  [unwired: 9 in]
    }
    frame 174 {
      # "LDX abs"
      n703 = call "CPU_MEM_read_mem_16.vi"("registers"=w977) -> ("value"=w975:u16, "registers"=w976:T1)  [unwired: 9 in]
      n704 = call "CPU_MEM_read_mem.vi"("address"=w975) -> ("value out"=w978:u8)  [unwired: 10 in]
      n705 = Bundle By Name(cluster=w976, "X"=w978) -> (w980:T1)
      n706 = call "CPU_P_update_ZN.vi"("value"=w978, "registers"=w980) -> ("registers"=w979:T1)  [unwired: 9 in]
    }
    frame 176 {
      # "BCS"
      n707 = call "OC_Branch_core.vi"("if set/clear"=TRUE, "flag"=enum8{"C", "Z", "I", "D", "B", "V", "N"}."C", "registers"=w982) -> ("registers"=w981:T1)  [unwired: 8 in]
    }
    frame 177 {
      # "LDA ind Y"
      n708 = Unbundle By Name(w993) -> ("PC"=w994:u16, "Y"=w988:u8)
      n709 = call "CPU_PC_inc.vi"("registers"=w993) -> ("registers"=w986:T1)  [unwired: 10 in]
      n710 = call "CPU_MEM_read_mem.vi"("address"=w994) -> ("value out"=w987:u8)  [unwired: 10 in]
      n711 = call "OC_read_ind_core.vi"("base"=w987) -> ("addr"=w985:u16)  [unwired: 10 in]
      n712 = Add(x=w985, y=w988) -> (x+y=w989:u16)
      n713 = call "CPU_MEM_read_mem.vi"("address"=w989) -> ("value out"=w990:u8)  [unwired: 10 in]
      n714 = Bundle By Name(cluster=w986, "A"=w990) -> (w992:T1)
      n715 = call "CPU_P_update_ZN.vi"("value"=w990, "registers"=w992) -> ("registers"=w991:T1)  [unwired: 9 in]
    }
    frame 180 {
      # "LDY zp X"
      n716 = Unbundle By Name(w1003) -> ("PC"=w1004:u16, "X"=w1002:u8)
      n717 = call "CPU_PC_inc.vi"("registers"=w1003) -> ("registers"=w999:T1)  [unwired: 10 in]
      n718 = call "CPU_MEM_read_mem.vi"("address"=w1004) -> ("value out"=w997:u8)  [unwired: 10 in]
      n719 = Add(x=w1002, y=w997) -> (x+y=w1000:u8)
      n720 = To Unsigned Word Integer(number=w1000) -> (unsigned 16bit integer=w996:u16)
      n721 = call "CPU_MEM_read_mem.vi"("address"=w996) -> ("value out"=w995:u8)  [unwired: 10 in]
      n722 = Bundle By Name(cluster=w999, "Y"=w995) -> (w998:T1)
      n723 = call "CPU_P_update_ZN.vi"("value"=w995, "registers"=w998) -> ("registers"=w1001:T1)  [unwired: 9 in]
    }
    frame 181 {
      # "LDA zp X"
      n724 = Unbundle By Name(w1013) -> ("PC"=w1014:u16, "X"=w1012:u8)
      n725 = call "CPU_PC_inc.vi"("registers"=w1013) -> ("registers"=w1009:T1)  [unwired: 10 in]
      n726 = call "CPU_MEM_read_mem.vi"("address"=w1014) -> ("value out"=w1007:u8)  [unwired: 10 in]
      n727 = Add(x=w1012, y=w1007) -> (x+y=w1010:u8)
      n728 = To Unsigned Word Integer(number=w1010) -> (unsigned 16bit integer=w1006:u16)
      n729 = call "CPU_MEM_read_mem.vi"("address"=w1006) -> ("value out"=w1005:u8)  [unwired: 10 in]
      n730 = Bundle By Name(cluster=w1009, "A"=w1005) -> (w1008:T1)
      n731 = call "CPU_P_update_ZN.vi"("value"=w1005, "registers"=w1008) -> ("registers"=w1011:T1)  [unwired: 9 in]
    }
    frame 182 {
      # "LDX addr Y"
      n732 = Unbundle By Name(w1023) -> ("PC"=w1024:u16, "Y"=w1017:u8)
      n733 = call "CPU_PC_inc.vi"("registers"=w1023) -> ("registers"=w1019:T1)  [unwired: 10 in]
      n734 = call "CPU_MEM_read_mem.vi"("address"=w1024) -> ("value out"=w1016:u8)  [unwired: 10 in]
      n735 = Add(x=w1016, y=w1017) -> (x+y=w1018:u8)
      n736 = To Unsigned Word Integer(number=w1018) -> (unsigned 16bit integer=w1015:u16)
      n737 = call "CPU_MEM_read_mem.vi"("address"=w1015) -> ("value out"=w1020:u8)  [unwired: 10 in]
      n738 = Bundle By Name(cluster=w1019, "X"=w1020) -> (w1022:T1)
      n739 = call "CPU_P_update_ZN.vi"("value"=w1020, "registers"=w1022) -> ("registers"=w1021:T1)  [unwired: 9 in]
    }
    frame 184 {
      # "CLV"
      n740 = call "CPU_P_update.vi"("flag"=enum8{"C", "Z", "I", "D", "B", "V", "N"}."V", "Value"=FALSE, "registers"=w1028) -> ("registers"=w1025:T1)  [unwired: 8 in]
    }
    frame 185 {
      # "LDA abs Y"
      n741 = Unbundle By Name(w1031) -> ("Y"=w1033:u8)
      n742 = call "CPU_MEM_read_mem_16.vi"("registers"=w1031) -> ("value"=w1029:u16, "registers"=w1030:T1)  [unwired: 9 in]
      n743 = Add(x=w1029, y=w1033) -> (x+y=w1034:u16)
      n744 = call "CPU_MEM_read_mem.vi"("address"=w1034) -> ("value out"=w1032:u8)  [unwired: 10 in]
      n745 = Bundle By Name(cluster=w1030, "A"=w1032) -> (w1036:T1)
      n746 = call "CPU_P_update_ZN.vi"("value"=w1032, "registers"=w1036) -> ("registers"=w1035:T1)  [unwired: 9 in]
    }
    frame 186 {
      # "TSX"
      n747 = Unbundle By Name(w1040) -> ("SP"=w1038:u8)
      n748 = Bundle By Name(cluster=w1040, "X"=w1038) -> (w1039:T1)
      n749 = call "CPU_P_update_ZN.vi"("value"=w1038, "registers"=w1039) -> ("registers"=w1037:T1)  [unwired: 9 in]
    }
    frame 188 {
      # "LDY abs X"
      n750 = Unbundle By Name(w1043) -> ("X"=w1045:u8)
      n751 = call "CPU_MEM_read_mem_16.vi"("registers"=w1043) -> ("value"=w1041:u16, "registers"=w1042:T1)  [unwired: 9 in]
      n752 = Add(x=w1041, y=w1045) -> (x+y=w1046:u16)
      n753 = call "CPU_MEM_read_mem.vi"("address"=w1046) -> ("value out"=w1044:u8)  [unwired: 10 in]
      n754 = Bundle By Name(cluster=w1042, "Y"=w1044) -> (w1048:T1)
      n755 = call "CPU_P_update_ZN.vi"("value"=w1044, "registers"=w1048) -> ("registers"=w1047:T1)  [unwired: 9 in]
    }
    frame 189 {
      # "LDA abs X"
      n756 = Unbundle By Name(w1051) -> ("X"=w1052:u8)
      n757 = call "CPU_MEM_read_mem_16.vi"("registers"=w1051) -> ("value"=w1049:u16, "registers"=w1050:T1)  [unwired: 9 in]
      n758 = Add(x=w1049, y=w1052) -> (x+y=w1053:u16)
      n759 = call "CPU_MEM_read_mem.vi"("address"=w1053) -> ("value out"=w1054:u8)  [unwired: 10 in]
      n760 = Bundle By Name(cluster=w1050, "A"=w1054) -> (w1056:T1)
      n761 = call "CPU_P_update_ZN.vi"("value"=w1054, "registers"=w1056) -> ("registers"=w1055:T1)  [unwired: 9 in]
    }
    frame 190 {
      # "LDX abs Y"
      n762 = Unbundle By Name(w1059) -> ("Y"=w1061:u8)
      n763 = call "CPU_MEM_read_mem_16.vi"("registers"=w1059) -> ("value"=w1057:u16, "registers"=w1058:T1)  [unwired: 9 in]
      n764 = Add(x=w1057, y=w1061) -> (x+y=w1062:u16)
      n765 = call "CPU_MEM_read_mem.vi"("address"=w1062) -> ("value out"=w1060:u8)  [unwired: 10 in]
      n766 = Bundle By Name(cluster=w1058, "X"=w1060) -> (w1064:T1)
      n767 = call "CPU_P_update_ZN.vi"("value"=w1060, "registers"=w1064) -> ("registers"=w1063:T1)  [unwired: 9 in]
    }
    frame 192 {
      # "CPY imm"
      n768 = Unbundle By Name(w1065) -> ("PC"=w1074:u16, "Y"=w1073:u8)
      n769 = call "CPU_PC_inc.vi"("registers"=w1065) -> ("registers"=w1066:T1)  [unwired: 10 in]
      n770 = call "CPU_MEM_read_mem.vi"("address"=w1074) -> ("value out"=w1072:u8)  [unwired: 10 in]
      n771 = Subtract(x=w1073, y=w1072) -> (x-y=w1067:u8)
      n772 = Greater Or Equal?(x=w1073, y=w1072) -> (x >= y?=w1070:bool)
      n773 = call "CPU_P_update.vi"("flag"=enum8{"C", "Z", "I", "D", "B", "V", "N"}."C", "Value"=w1070, "registers"=w1066) -> ("registers"=w1069:T1)  [unwired: 8 in]
      n774 = call "CPU_P_update_ZN.vi"("value"=w1067, "registers"=w1069) -> ("registers"=w1068:T1)  [unwired: 9 in]
    }
    frame 193 {
      # "CMP indx"
      n775 = Unbundle By Name(w1087) -> ("PC"=w1088:u16, "A"=w1086:u8, "X"=w1077:u8)
      n776 = call "CPU_PC_inc.vi"("registers"=w1087) -> ("registers"=w1085:T1)  [unwired: 10 in]
      n777 = call "CPU_MEM_read_mem.vi"("address"=w1088) -> ("value out"=w1078:u8)  [unwired: 10 in]
      n778 = Add(x=w1078, y=w1077) -> (x+y=w1076:u8)
      n779 = call "OC_read_ind_core.vi"("base"=w1076) -> ("addr"=w1075:u16)  [unwired: 10 in]
      n780 = call "CPU_MEM_read_mem.vi"("address"=w1075) -> ("value out"=w1079:u8)  [unwired: 10 in]
      n781 = Subtract(x=w1086, y=w1079) -> (x-y=w1080:u8)
      n782 = Greater Or Equal?(x=w1086, y=w1079) -> (x >= y?=w1083:bool)
      n783 = call "CPU_P_update.vi"("flag"=enum8{"C", "Z", "I", "D", "B", "V", "N"}."C", "Value"=w1083, "registers"=w1085) -> ("registers"=w1082:T1)  [unwired: 8 in]
      n784 = call "CPU_P_update_ZN.vi"("value"=w1080, "registers"=w1082) -> ("registers"=w1081:T1)  [unwired: 9 in]
    }
    frame 196 {
      # "CPY zp"
      n785 = Unbundle By Name(w1099) -> ("PC"=w1100:u16, "Y"=w1098:u8)
      n786 = call "CPU_PC_inc.vi"("registers"=w1099) -> ("registers"=w1097:T1)  [unwired: 10 in]
      n787 = call "CPU_MEM_read_mem.vi"("address"=w1100) -> ("value out"=w1091:u8)  [unwired: 10 in]
      n788 = To Unsigned Word Integer(number=w1091) -> (unsigned 16bit integer=w1089:u16)
      n789 = call "CPU_MEM_read_mem.vi"("address"=w1089) -> ("value out"=w1090:u8)  [unwired: 10 in]
      n790 = Subtract(x=w1098, y=w1090) -> (x-y=w1092:u8)
      n791 = Greater Or Equal?(x=w1098, y=w1090) -> (x >= y?=w1095:bool)
      n792 = call "CPU_P_update.vi"("flag"=enum8{"C", "Z", "I", "D", "B", "V", "N"}."C", "Value"=w1095, "registers"=w1097) -> ("registers"=w1094:T1)  [unwired: 8 in]
      n793 = call "CPU_P_update_ZN.vi"("value"=w1092, "registers"=w1094) -> ("registers"=w1093:T1)  [unwired: 9 in]
    }
    frame 197 {
      # "CMP zp"
      n794 = Unbundle By Name(w1111) -> ("PC"=w1112:u16, "A"=w1110:u8)
      n795 = call "CPU_PC_inc.vi"("registers"=w1111) -> ("registers"=w1109:T1)  [unwired: 10 in]
      n796 = call "CPU_MEM_read_mem.vi"("address"=w1112) -> ("value out"=w1103:u8)  [unwired: 10 in]
      n797 = To Unsigned Word Integer(number=w1103) -> (unsigned 16bit integer=w1101:u16)
      n798 = call "CPU_MEM_read_mem.vi"("address"=w1101) -> ("value out"=w1102:u8)  [unwired: 10 in]
      n799 = Subtract(x=w1110, y=w1102) -> (x-y=w1104:u8)
      n800 = Greater Or Equal?(x=w1110, y=w1102) -> (x >= y?=w1107:bool)
      n801 = call "CPU_P_update.vi"("flag"=enum8{"C", "Z", "I", "D", "B", "V", "N"}."C", "Value"=w1107, "registers"=w1109) -> ("registers"=w1106:T1)  [unwired: 8 in]
      n802 = call "CPU_P_update_ZN.vi"("value"=w1104, "registers"=w1106) -> ("registers"=w1105:T1)  [unwired: 9 in]
    }
    frame 198 {
      # "DEC zp"
      n803 = Unbundle By Name(w1115) -> ("PC"=w1121:u16)
      n804 = call "CPU_PC_inc.vi"("registers"=w1115) -> ("registers"=w1114:T1)  [unwired: 10 in]
      n805 = call "CPU_MEM_read_mem.vi"("address"=w1121) -> ("value out"=w1120:u8)  [unwired: 10 in]
      n806 = To Unsigned Word Integer(number=w1120) -> (unsigned 16bit integer=w1117:u16)
      n807 = call "CPU_MEM_read_mem.vi"("address"=w1117) -> ("value out"=w1118:u8)  [unwired: 10 in]
      n808 = Subtract(x=w1118, y=u8 1) -> (x-y=w1116:u8)
      n809 = call "CPU_MEM_write_mem.vi"("value"=w1116, "address"=w1117) -> ()  [unwired: 10 in]
      n810 = call "CPU_P_update_ZN.vi"("value"=w1116, "registers"=w1114) -> ("registers"=w1113:T1)  [unwired: 9 in]
    }
    frame 200 {
      # "INY"
      n811 = Unbundle By Name(w1126) -> ("Y"=w1124:u8)
      n812 = Increment(x=w1124) -> (x+1=w1123:u8)
      n813 = Bundle By Name(cluster=w1126, "Y"=w1123) -> (w1125:T1)
      n814 = call "CPU_P_update_ZN.vi"("value"=w1123, "registers"=w1125) -> ("registers"=w1122:T1)  [unwired: 9 in]
    }
    frame 201 {
      # "CMP imm"
      n815 = Unbundle By Name(w1127) -> ("PC"=w1136:u16, "A"=w1135:u8)
      n816 = call "CPU_PC_inc.vi"("registers"=w1127) -> ("registers"=w1128:T1)  [unwired: 10 in]
      n817 = call "CPU_MEM_read_mem.vi"("address"=w1136) -> ("value out"=w1134:u8)  [unwired: 10 in]
      n818 = Subtract(x=w1135, y=w1134) -> (x-y=w1129:u8)
      n819 = Greater Or Equal?(x=w1135, y=w1134) -> (x >= y?=w1132:bool)
      n820 = call "CPU_P_update.vi"("flag"=enum8{"C", "Z", "I", "D", "B", "V", "N"}."C", "Value"=w1132, "registers"=w1128) -> ("registers"=w1131:T1)  [unwired: 8 in]
      n821 = call "CPU_P_update_ZN.vi"("value"=w1129, "registers"=w1131) -> ("registers"=w1130:T1)  [unwired: 9 in]
    }
    frame 202 {
      # "DEX"
      n822 = Unbundle By Name(w1141) -> ("X"=w1139:u8)
      n823 = Decrement(x=w1139) -> (x-1=w1138:u8)
      n824 = Bundle By Name(cluster=w1141, "X"=w1138) -> (w1140:T1)
      n825 = call "CPU_P_update_ZN.vi"("value"=w1138, "registers"=w1140) -> ("registers"=w1137:T1)  [unwired: 9 in]
    }
    frame 204 {
      # "CPY abs"
      n826 = Unbundle By Name(w1144) -> ("Y"=w1151:u8)
      n827 = call "CPU_MEM_read_mem_16.vi"("registers"=w1144) -> ("value"=w1142:u16, "registers"=w1143:T1)  [unwired: 9 in]
      n828 = call "CPU_MEM_read_mem.vi"("address"=w1142) -> ("value out"=w1145:u8)  [unwired: 10 in]
      n829 = Subtract(x=w1151, y=w1145) -> (x-y=w1146:u8)
      n830 = Greater Or Equal?(x=w1151, y=w1145) -> (x >= y?=w1149:bool)
      n831 = call "CPU_P_update.vi"("flag"=enum8{"C", "Z", "I", "D", "B", "V", "N"}."C", "Value"=w1149, "registers"=w1143) -> ("registers"=w1148:T1)  [unwired: 8 in]
      n832 = call "CPU_P_update_ZN.vi"("value"=w1146, "registers"=w1148) -> ("registers"=w1147:T1)  [unwired: 9 in]
    }
    frame 205 {
      # "CMP abs"
      n833 = Unbundle By Name(w1154) -> ("A"=w1161:u8)
      n834 = call "CPU_MEM_read_mem_16.vi"("registers"=w1154) -> ("value"=w1152:u16, "registers"=w1153:T1)  [unwired: 9 in]
      n835 = call "CPU_MEM_read_mem.vi"("address"=w1152) -> ("value out"=w1155:u8)  [unwired: 10 in]
      n836 = Subtract(x=w1161, y=w1155) -> (x-y=w1156:u8)
      n837 = Greater Or Equal?(x=w1161, y=w1155) -> (x >= y?=w1159:bool)
      n838 = call "CPU_P_update.vi"("flag"=enum8{"C", "Z", "I", "D", "B", "V", "N"}."C", "Value"=w1159, "registers"=w1153) -> ("registers"=w1158:T1)  [unwired: 8 in]
      n839 = call "CPU_P_update_ZN.vi"("value"=w1156, "registers"=w1158) -> ("registers"=w1157:T1)  [unwired: 9 in]
    }
    frame 206 {
      # "DEC abs"
      n840 = call "CPU_MEM_read_mem_16.vi"("registers"=w1164) -> ("value"=w1162:u16, "registers"=w1163:T1)  [unwired: 9 in]
      n841 = call "CPU_MEM_read_mem.vi"("address"=w1162) -> ("value out"=w1167:u8)  [unwired: 10 in]
      n842 = Subtract(x=w1167, y=u8 1) -> (x-y=w1165:u8)
      n843 = call "CPU_MEM_write_mem.vi"("value"=w1165, "address"=w1162) -> ()  [unwired: 10 in]
      n844 = call "CPU_P_update_ZN.vi"("value"=w1165, "registers"=w1163) -> ("registers"=w1168:T1)  [unwired: 9 in]
    }
    frame 208 {
      # "BNE"
      n845 = call "OC_Branch_core.vi"("if set/clear"=FALSE, "flag"=enum8{"C", "Z", "I", "D", "B", "V", "N"}."Z", "registers"=w1170) -> ("registers"=w1169:T1)  [unwired: 8 in]
    }
    frame 209 {
      # "CMP indy"
      n846 = Unbundle By Name(w1185) -> ("PC"=w1186:u16, "A"=w1184:u8, "Y"=w1173:u8)
      n847 = call "CPU_PC_inc.vi"("registers"=w1185) -> ("registers"=w1183:T1)  [unwired: 10 in]
      n848 = call "CPU_MEM_read_mem.vi"("address"=w1186) -> ("value out"=w1176:u8)  [unwired: 10 in]
      n849 = call "OC_read_ind_core.vi"("base"=w1176) -> ("addr"=w1175:u16)  [unwired: 10 in]
      n850 = Add(x=w1175, y=w1173) -> (x+y=w1174:u16)
      n851 = call "CPU_MEM_read_mem.vi"("address"=w1174) -> ("value out"=w1177:u8)  [unwired: 10 in]
      n852 = Subtract(x=w1184, y=w1177) -> (x-y=w1178:u8)
      n853 = Greater Or Equal?(x=w1184, y=w1177) -> (x >= y?=w1181:bool)
      n854 = call "CPU_P_update.vi"("flag"=enum8{"C", "Z", "I", "D", "B", "V", "N"}."C", "Value"=w1181, "registers"=w1183) -> ("registers"=w1180:T1)  [unwired: 8 in]
      n855 = call "CPU_P_update_ZN.vi"("value"=w1178, "registers"=w1180) -> ("registers"=w1179:T1)  [unwired: 9 in]
    }
    frame 213 {
      # "CMP zpx"
      n856 = Unbundle By Name(w1199) -> ("PC"=w1200:u16, "A"=w1198:u8, "X"=w1189:u8)
      n857 = call "CPU_PC_inc.vi"("registers"=w1199) -> ("registers"=w1197:T1)  [unwired: 10 in]
      n858 = call "CPU_MEM_read_mem.vi"("address"=w1200) -> ("value out"=w1190:u8)  [unwired: 10 in]
      n859 = Add(x=w1190, y=w1189) -> (x+y=w1188:u8)
      n860 = To Unsigned Word Integer(number=w1188) -> (unsigned 16bit integer=w1187:u16)
      n861 = call "CPU_MEM_read_mem.vi"("address"=w1187) -> ("value out"=w1191:u8)  [unwired: 10 in]
      n862 = Subtract(x=w1198, y=w1191) -> (x-y=w1192:u8)
      n863 = Greater Or Equal?(x=w1198, y=w1191) -> (x >= y?=w1195:bool)
      n864 = call "CPU_P_update.vi"("flag"=enum8{"C", "Z", "I", "D", "B", "V", "N"}."C", "Value"=w1195, "registers"=w1197) -> ("registers"=w1194:T1)  [unwired: 8 in]
      n865 = call "CPU_P_update_ZN.vi"("value"=w1192, "registers"=w1194) -> ("registers"=w1193:T1)  [unwired: 9 in]
    }
    frame 214 {
      # "DEC zp X"
      n866 = Unbundle By Name(w1206) -> ("PC"=w1211:u16, "X"=w1203:u8)
      n867 = call "CPU_PC_inc.vi"("registers"=w1206) -> ("registers"=w1205:T1)  [unwired: 10 in]
      n868 = call "CPU_MEM_read_mem.vi"("address"=w1211) -> ("value out"=w1202:u8)  [unwired: 10 in]
      n869 = Add(x=w1202, y=w1203) -> (x+y=w1201:u8)
      n870 = To Unsigned Word Integer(number=w1201) -> (unsigned 16bit integer=w1208:u16)
      n871 = call "CPU_MEM_read_mem.vi"("address"=w1208) -> ("value out"=w1209:u8)  [unwired: 10 in]
      n872 = Subtract(x=w1209, y=u8 1) -> (x-y=w1207:u8)
      n873 = call "CPU_MEM_write_mem.vi"("value"=w1207, "address"=w1208) -> ()  [unwired: 10 in]
      n874 = call "CPU_P_update_ZN.vi"("value"=w1207, "registers"=w1205) -> ("registers"=w1204:T1)  [unwired: 9 in]
    }
    frame 216 {
      # "CLD"
      n875 = call "CPU_P_update.vi"("flag"=enum8{"C", "Z", "I", "D", "B", "V", "N"}."D", "Value"=FALSE, "registers"=w1213) -> ("registers"=w1212:T1)  [unwired: 8 in]
    }
    frame 217 {
      # "CMP abs Y"
      n876 = Unbundle By Name(w1220) -> ("A"=w1217:u8, "Y"=w1216:u8)
      n877 = call "CPU_MEM_read_mem_16.vi"("registers"=w1220) -> ("value"=w1218:u16, "registers"=w1219:T1)  [unwired: 9 in]
      n878 = Add(x=w1218, y=w1216) -> (x+y=w1226:u16)
      n879 = call "CPU_MEM_read_mem.vi"("address"=w1226) -> ("value out"=w1222:u8)  [unwired: 10 in]
      n880 = Subtract(x=w1217, y=w1222) -> (x-y=w1225:u8)
      n881 = Greater Or Equal?(x=w1217, y=w1222) -> (x >= y?=w1221:bool)
      n882 = call "CPU_P_update.vi"("flag"=enum8{"C", "Z", "I", "D", "B", "V", "N"}."C", "Value"=w1221, "registers"=w1219) -> ("registers"=w1223:T1)  [unwired: 8 in]
      n883 = call "CPU_P_update_ZN.vi"("value"=w1225, "registers"=w1223) -> ("registers"=w1227:T1)  [unwired: 9 in]
    }
    frame 221 {
      # "CMP absx"
      n884 = call "CPU_MEM_read_mem_16.vi"("registers"=w1230) -> ("value"=w1228:u16, "registers"=w1229:T1)  [unwired: 9 in]
      n885 = Unbundle By Name(w1230) -> ("A"=w1239:u8, "X"=w1232:u8)
      n886 = Add(x=w1228, y=w1232) -> (x+y=w1231:u16)
      n887 = call "CPU_MEM_read_mem.vi"("address"=w1231) -> ("value out"=w1233:u8)  [unwired: 10 in]
      n888 = Subtract(x=w1239, y=w1233) -> (x-y=w1234:u8)
      n889 = Greater Or Equal?(x=w1239, y=w1233) -> (x >= y?=w1237:bool)
      n890 = call "CPU_P_update.vi"("flag"=enum8{"C", "Z", "I", "D", "B", "V", "N"}."C", "Value"=w1237, "registers"=w1229) -> ("registers"=w1236:T1)  [unwired: 8 in]
      n891 = call "CPU_P_update_ZN.vi"("value"=w1234, "registers"=w1236) -> ("registers"=w1235:T1)  [unwired: 9 in]
    }
    frame 222 {
      # "DEC abs X"
      n892 = Unbundle By Name(w1242) -> ("X"=w1243:u8)
      n893 = call "CPU_MEM_read_mem_16.vi"("registers"=w1242) -> ("value"=w1240:u16, "registers"=w1241:T1)  [unwired: 9 in]
      n894 = Add(x=w1240, y=w1243) -> (x+y=w1244:u16)
      n895 = call "CPU_MEM_read_mem.vi"("address"=w1244) -> ("value out"=w1247:u8)  [unwired: 10 in]
      n896 = Subtract(x=w1247, y=u8 1) -> (x-y=w1245:u8)
      n897 = call "CPU_MEM_write_mem.vi"("value"=w1245, "address"=w1244) -> ()  [unwired: 10 in]
      n898 = call "CPU_P_update_ZN.vi"("value"=w1245, "registers"=w1241) -> ("registers"=w1248:T1)  [unwired: 9 in]
    }
    frame 224 {
      # "CPX imm"
      n899 = Unbundle By Name(w1249) -> ("PC"=w1258:u16, "X"=w1257:u8)
      n900 = call "CPU_PC_inc.vi"("registers"=w1249) -> ("registers"=w1250:T1)  [unwired: 10 in]
      n901 = call "CPU_MEM_read_mem.vi"("address"=w1258) -> ("value out"=w1256:u8)  [unwired: 10 in]
      n902 = Subtract(x=w1257, y=w1256) -> (x-y=w1251:u8)
      n903 = Greater Or Equal?(x=w1257, y=w1256) -> (x >= y?=w1254:bool)
      n904 = call "CPU_P_update.vi"("flag"=enum8{"C", "Z", "I", "D", "B", "V", "N"}."C", "Value"=w1254, "registers"=w1250) -> ("registers"=w1253:T1)  [unwired: 8 in]
      n905 = call "CPU_P_update_ZN.vi"("value"=w1251, "registers"=w1253) -> ("registers"=w1252:T1)  [unwired: 9 in]
    }
    frame 225 {
      # "SBC indx"
      n906 = Unbundle By Name(w1267) -> ("PC"=w1265:u16, "X"=w1266:u8)
      n907 = call "CPU_PC_inc.vi"("registers"=w1267) -> ("registers"=w1261:T1)  [unwired: 10 in]
      n908 = call "CPU_MEM_read_mem.vi"("address"=w1265) -> ("value out"=w1264:u8)  [unwired: 10 in]
      n909 = Add(x=w1264, y=w1266) -> (x+y=w1263:u8)
      n910 = call "OC_read_ind_core.vi"("base"=w1263) -> ("addr"=w1262:u16)  [unwired: 10 in]
      n911 = call "CPU_MEM_read_mem.vi"("address"=w1262) -> ("value out"=w1259:u8)  [unwired: 10 in]
      n912 = call "OC_SBC_core.vi"("value"=w1259, "registers"=w1261) -> ("registers"=w1260:T1)  [unwired: 9 in]
    }
    frame 228 {
      # "CPX zp"
      n913 = call "CPU_PC_inc.vi"("registers"=w1278) -> ("registers"=w1276:T1)  [unwired: 10 in]
      n914 = Unbundle By Name(w1278) -> ("PC"=w1279:u16, "X"=w1277:u8)
      n915 = call "CPU_MEM_read_mem.vi"("address"=w1279) -> ("value out"=w1270:u8)  [unwired: 10 in]
      n916 = To Unsigned Word Integer(number=w1270) -> (unsigned 16bit integer=w1268:u16)
      n917 = call "CPU_MEM_read_mem.vi"("address"=w1268) -> ("value out"=w1269:u8)  [unwired: 10 in]
      n918 = Subtract(x=w1277, y=w1269) -> (x-y=w1271:u8)
      n919 = Greater Or Equal?(x=w1277, y=w1269) -> (x >= y?=w1274:bool)
      n920 = call "CPU_P_update.vi"("flag"=enum8{"C", "Z", "I", "D", "B", "V", "N"}."C", "Value"=w1274, "registers"=w1276) -> ("registers"=w1273:T1)  [unwired: 8 in]
      n921 = call "CPU_P_update_ZN.vi"("value"=w1271, "registers"=w1273) -> ("registers"=w1272:T1)  [unwired: 9 in]
    }
    frame 229 {
      # "SBC zp"
      # "ADC"
      n922 = Unbundle By Name(w1285) -> ("PC"=w1286:u16)
      n923 = call "CPU_PC_inc.vi"("registers"=w1285) -> ("registers"=w1284:T1)  [unwired: 10 in]
      n924 = call "CPU_MEM_read_mem.vi"("address"=w1286) -> ("value out"=w1282:u8)  [unwired: 10 in]
      n925 = To Unsigned Word Integer(number=w1282) -> (unsigned 16bit integer=w1280:u16)
      n926 = call "CPU_MEM_read_mem.vi"("address"=w1280) -> ("value out"=w1281:u8)  [unwired: 10 in]
      n927 = call "OC_SBC_core.vi"("value"=w1281, "registers"=w1284) -> ("registers"=w1283:T1)  [unwired: 9 in]
    }
    frame 245 {
      # "SBC zp X"
      # "ADC"
      n928 = Unbundle By Name(w1294) -> ("PC"=w1295:u16, "X"=w1287:u8)
      n929 = call "CPU_PC_inc.vi"("registers"=w1294) -> ("registers"=w1293:T1)  [unwired: 10 in]
      n930 = call "CPU_MEM_read_mem.vi"("address"=w1295) -> ("value out"=w1291:u8)  [unwired: 10 in]
      n931 = Add(x=w1291, y=w1287) -> (x+y=w1288:u8)
      n932 = To Unsigned Word Integer(number=w1288) -> (unsigned 16bit integer=w1289:u16)
      n933 = call "CPU_MEM_read_mem.vi"("address"=w1289) -> ("value out"=w1290:u8)  [unwired: 10 in]
      n934 = call "OC_SBC_core.vi"("value"=w1290, "registers"=w1293) -> ("registers"=w1292:T1)  [unwired: 9 in]
    }
    frame 230 {
      # "INC zp"
      n935 = Unbundle By Name(w1296) -> ("PC"=w1302:u16)
      n936 = call "CPU_MEM_read_mem.vi"("address"=w1302) -> ("value out"=w1301:u8)  [unwired: 10 in]
      n937 = To Unsigned Word Integer(number=w1301) -> (unsigned 16bit integer=w1298:u16)
      n938 = call "CPU_MEM_read_mem.vi"("address"=w1298) -> ("value out"=w1299:u8)  [unwired: 10 in]
      n939 = Add(x=w1299, y=u8 1) -> (x+y=w1297:u8)
      n940 = call "CPU_MEM_write_mem.vi"("value"=w1297, "address"=w1298) -> ()  [unwired: 10 in]
      n941 = call "CPU_P_update_ZN.vi"("value"=w1297, "registers"=w1296) -> ("registers"=w1303:T1)  [unwired: 9 in]
      n942 = call "CPU_PC_inc.vi"("registers"=w1303) -> ("registers"=w1304:T1)  [unwired: 10 in]
    }
    frame 232 {
      # "INX"
      n943 = Unbundle By Name(w1309) -> ("X"=w1307:u8)
      n944 = Increment(x=w1307) -> (x+1=w1306:u8)
      n945 = Bundle By Name(cluster=w1309, "X"=w1306) -> (w1308:T1)
      n946 = call "CPU_P_update_ZN.vi"("value"=w1306, "registers"=w1308) -> ("registers"=w1305:T1)  [unwired: 9 in]
    }
    frame 233 {
      # "SBC imm"
      # "ADC"
      n947 = Unbundle By Name(w1313) -> ("PC"=w1314:u16)
      n948 = call "CPU_PC_inc.vi"("registers"=w1313) -> ("registers"=w1312:T1)  [unwired: 10 in]
      n949 = call "CPU_MEM_read_mem.vi"("address"=w1314) -> ("value out"=w1310:u8)  [unwired: 10 in]
      n950 = call "OC_SBC_core.vi"("value"=w1310, "registers"=w1312) -> ("registers"=w1311:T1)  [unwired: 9 in]
    }
    frame 234 {
      # "NOP"
    }
    frame 236 {
      # "CPX abs"
      n951 = Unbundle By Name(w1318) -> ("X"=w1325:u8)
      n952 = call "CPU_MEM_read_mem_16.vi"("registers"=w1318) -> ("value"=w1316:u16, "registers"=w1317:T1)  [unwired: 9 in]
      n953 = call "CPU_MEM_read_mem.vi"("address"=w1316) -> ("value out"=w1319:u8)  [unwired: 10 in]
      n954 = Subtract(x=w1325, y=w1319) -> (x-y=w1320:u8)
      n955 = Greater Or Equal?(x=w1325, y=w1319) -> (x >= y?=w1323:bool)
      n956 = call "CPU_P_update.vi"("flag"=enum8{"C", "Z", "I", "D", "B", "V", "N"}."C", "Value"=w1323, "registers"=w1317) -> ("registers"=w1322:T1)  [unwired: 8 in]
      n957 = call "CPU_P_update_ZN.vi"("value"=w1320, "registers"=w1322) -> ("registers"=w1321:T1)  [unwired: 9 in]
    }
    frame 237 {
      # "SBC abs"
      # "ADC"
      n958 = call "CPU_MEM_read_mem_16.vi"("registers"=w1328) -> ("value"=w1326:u16, "registers"=w1327:T1)  [unwired: 9 in]
      n959 = call "CPU_MEM_read_mem.vi"("address"=w1326) -> ("value out"=w1329:u8)  [unwired: 10 in]
      n960 = call "OC_SBC_core.vi"("value"=w1329, "registers"=w1327) -> ("registers"=w1330:T1)  [unwired: 9 in]
    }
    frame 253 {
      # "SBC abs X"
      # "ADC"
      n961 = call "CPU_MEM_read_mem_16.vi"("registers"=w1333) -> ("value"=w1331:u16, "registers"=w1332:T1)  [unwired: 9 in]
      n962 = Unbundle By Name(w1333) -> ("X"=w1334:u8)
      n963 = Add(x=w1331, y=w1334) -> (x+y=w1335:u16)
      n964 = call "CPU_MEM_read_mem.vi"("address"=w1335) -> ("value out"=w1336:u8)  [unwired: 10 in]
      n965 = call "OC_SBC_core.vi"("value"=w1336, "registers"=w1332) -> ("registers"=w1337:T1)  [unwired: 9 in]
    }
    frame 249 {
      # "SBC abs Y"
      # "ADC"
      n966 = call "CPU_MEM_read_mem_16.vi"("registers"=w1340) -> ("value"=w1338:u16, "registers"=w1339:T1)  [unwired: 9 in]
      n967 = Unbundle By Name(w1340) -> ("Y"=w1341:u8)
      n968 = Add(x=w1338, y=w1341) -> (x+y=w1342:u16)
      n969 = call "CPU_MEM_read_mem.vi"("address"=w1342) -> ("value out"=w1343:u8)  [unwired: 10 in]
      n970 = call "OC_SBC_core.vi"("value"=w1343, "registers"=w1339) -> ("registers"=w1344:T1)  [unwired: 9 in]
    }
    frame 238 {
      # "INC abs"
      n971 = call "CPU_MEM_read_mem_16.vi"("registers"=w1347) -> ("value"=w1345:u16, "registers"=w1346:T1)  [unwired: 9 in]
      n972 = call "CPU_MEM_read_mem.vi"("address"=w1345) -> ("value out"=w1350:u8)  [unwired: 10 in]
      n973 = Increment(x=w1350) -> (x+1=w1348:u8)
      n974 = call "CPU_MEM_write_mem.vi"("value"=w1348, "address"=w1345) -> ()  [unwired: 10 in]
      n975 = call "CPU_P_update_ZN.vi"("value"=w1348, "registers"=w1346) -> ("registers"=w1349:T1)  [unwired: 9 in]
    }
    frame 240 {
      # "BEQ"
      n976 = call "OC_Branch_core.vi"("if set/clear"=TRUE, "flag"=enum8{"C", "Z", "I", "D", "B", "V", "N"}."Z", "registers"=w1354) -> ("registers"=w1353:T1)  [unwired: 8 in]
    }
    frame 241 {
      # "SBC indy"
      n977 = Unbundle By Name(w1363) -> ("PC"=w1362:u16, "Y"=w1357:u8)
      n978 = call "CPU_PC_inc.vi"("registers"=w1363) -> ("registers"=w1361:T1)  [unwired: 10 in]
      n979 = call "CPU_MEM_read_mem.vi"("address"=w1362) -> ("value out"=w1358:u8)  [unwired: 10 in]
      n980 = call "OC_read_ind_core.vi"("base"=w1358) -> ("addr"=w1356:u16)  [unwired: 10 in]
      n981 = Add(x=w1356, y=w1357) -> (x+y=w1355:u16)
      n982 = call "CPU_MEM_read_mem.vi"("address"=w1355) -> ("value out"=w1359:u8)  [unwired: 10 in]
      n983 = call "OC_SBC_core.vi"("value"=w1359, "registers"=w1361) -> ("registers"=w1360:T1)  [unwired: 9 in]
    }
    frame 246 {
      # "INC zp X"
      n984 = Unbundle By Name(w1367) -> ("PC"=w1372:u16, "X"=w1366:u8)
      n985 = call "CPU_MEM_read_mem.vi"("address"=w1372) -> ("value out"=w1365:u8)  [unwired: 10 in]
      n986 = Add(x=w1365, y=w1366) -> (x+y=w1364:u8)
      n987 = To Unsigned Word Integer(number=w1364) -> (unsigned 16bit integer=w1369:u16)
      n988 = call "CPU_MEM_read_mem.vi"("address"=w1369) -> ("value out"=w1370:u8)  [unwired: 10 in]
      n989 = Add(x=w1370, y=u8 1) -> (x+y=w1368:u8)
      n990 = call "CPU_MEM_write_mem.vi"("value"=w1368, "address"=w1369) -> ()  [unwired: 10 in]
      n991 = call "CPU_P_update_ZN.vi"("value"=w1368, "registers"=w1367) -> ("registers"=w1373:T1)  [unwired: 9 in]
      n992 = call "CPU_PC_inc.vi"("registers"=w1373) -> ("registers"=w1374:T1)  [unwired: 10 in]
    }
    frame 248 {
      # "SED"
      n993 = call "CPU_P_update.vi"("flag"=enum8{"C", "Z", "I", "D", "B", "V", "N"}."D", "Value"=TRUE, "registers"=w1376) -> ("registers"=w1375:T1)  [unwired: 8 in]
    }
    frame 254 {
      # "INC abs X"
      n994 = Unbundle By Name(w1381) -> ("X"=w1386:u8)
      n995 = call "CPU_MEM_read_mem_16.vi"("registers"=w1381) -> ("value"=w1379:u16, "registers"=w1380:T1)  [unwired: 9 in]
      n996 = Add(x=w1379, y=w1386) -> (x+y=w1385:u16)
      n997 = call "CPU_MEM_read_mem.vi"("address"=w1385) -> ("value out"=w1384:u8)  [unwired: 10 in]
      n998 = Increment(x=w1384) -> (x+1=w1382:u8)
      n999 = call "CPU_MEM_write_mem.vi"("value"=w1382, "address"=w1385) -> ()  [unwired: 10 in]
      n1000 = call "CPU_P_update_ZN.vi"("value"=w1382, "registers"=w1380) -> ("registers"=w1383:T1)  [unwired: 9 in]
    }
    frame Default {
      n1001 = Format Into String(format string="Error - OpCode not supported: 0x%02x ", w1390) -> (resulting string=w1389:string)  [unwired: 2 in, 1 out]
      n1002 = One Button Dialog(message=w1389) -> ()  [unwired: 1 in, 1 out]
    }
  }
  "registers" <- w3
  "error" <- w2
